vi "Tree_Sync_Hide items.vi"(7 "Action":T2, 8 "error in":errorcluster, 9 "Properties for Tree In":T1(array[cluster])=[{"Label"="AppBuilderCache", "Tag"="0.3.fa.AppBuilderCache", "Property Type"=enum."Base", "Indent"=0, "Can Read?"=FALSE, "Can Write?"=FALSE, "Is Read?"=FALSE, "Is Write?"=FALSE, "Inactive Parent?"=TRUE, "Unwired?"=FALSE}, {"Label"="Path", "Tag"="0.3.fa.AppBuilderCache:Path", "Property Type"=enum."Private", "Indent"=1, "Can Read?"=TRUE, "Can Write?"=FALSE, "Is Read?"=FALSE, "Is Write?"=FALSE, "Inactive Parent?"=FALSE, "Unwired?"=FALSE}, {"Label"="Application", "Tag"="1.2.80.Application", "Property Type"=enum."Base", "Indent"=0, "Can Read?"=FALSE, "Can Write?"=FALSE, "Is Read?"=FALSE, "Is Write?"=FALSE, "Inactive Parent?"=TRUE, "Unwired?"=FALSE}, {"Label"="Active", "Tag"="1.2.80.Application:Active", "Property Type"=enum."Base", "Indent"=1, "Can Read?"=FALSE, "Can Write?"=FALSE, "Is Read?"=FALSE, "Is Write?"=FALSE, "Inactive Parent?"=TRUE, "Unwired?"=FALSE}, {"Label"="Application", "Tag"="1.2.80.Application:Active:Application", "Property Type"=enum."Scripting", "Indent"=2, "Can Read?"=TRUE, "Can Write?"=FALSE, "Is Read?"=FALSE, "Is Write?"=FALSE, "Inactive Parent?"=FALSE, "Unwired?"=FALSE}, {"Label"="VI", "Tag"="2.2.46.Application:Active:VI", "Property Type"=enum."Scripting", "Indent"=2, "Can Read?"=TRUE, "Can Write?"=FALSE, "Is Read?"=FALSE, "Is Write?"=FALSE, "Inactive Parent?"=FALSE, "Unwired?"=FALSE}, {"Label"="All Contexts", "Tag"="3.3.68.Application:All Contexts", "Property Type"=enum."Private", "Indent"=1, "Can Read?"=TRUE, "Can Write?"=FALSE, "Is Read?"=FALSE, "Is Write?"=FALSE, "Inactive Parent?"=FALSE, "Unwired?"=FALSE}, {"Label"="All Libraries in Application Instance", "Tag"="4.1.cd.Application:All Libraries in Application Instance", "Property Type"=enum."Base", "Indent"=1, "Can Read?"=TRUE, "Can Write?"=FALSE, "Is Read?"=FALSE, "Is Write?"=FALSE, "Inactive Parent?"=FALSE, "Unwired?"=FALSE}, {"Label"="All System VIs in Memory", "Tag"="5.3.1e.Application:All System VIs in Memory", "Property Type"=enum."Private", "Indent"=1, "Can Read?"=TRUE, "Can Write?"=FALSE, "Is Read?"=FALSE, "Is Write?"=FALSE, "Inactive Parent?"=FALSE, "Unwired?"=FALSE}, {"Label"="All VIs In Memory", "Tag"="6.1.1c.Application:All VIs In Memory", "Property Type"=enum."Base", "Indent"=1, "Can Read?"=TRUE, "Can Write?"=FALSE, "Is Read?"=FALSE, "Is Write?"=FALSE, "Inactive Parent?"=FALSE, "Unwired?"=FALSE}, {"Label"="Assistants Use Strict Types Default", "Tag"="7.3.52.Application:Assistants Use Strict Types Default", "Property Type"=enum."Private", "Indent"=1, "Can Read?"=TRUE, "Can Write?"=TRUE, "Is Read?"=FALSE, "Is Write?"=FALSE, "Inactive Parent?"=FALSE, "Unwired?"=FALSE}, {"Label"="Auto-Route Wires", "Tag"="8.2.53.Application:Auto-Route Wires", "Property Type"=enum."Scripting", "Indent"=1, "Can Read?"=TRUE, "Can Write?"=TRUE, "Is Read?"=FALSE, "Is Write?"=FALSE, "Inactive Parent?"=FALSE, "Unwired?"=FALSE}, {"Label"="Available Environment Modes", "Tag"="9.3.dd.Application:Available Environment Modes", "Property Type"=enum."Private", "Indent"=1, "Can Read?"=TRUE, "Can Write?"=FALSE, "Is Read?"=FALSE, "Is Write?"=FALSE, "Inactive Parent?"=FALSE, "Unwired?"=FALSE}, {"Label"="Clipboard Mode", "Tag"="10.3.e4.Application:Clipboard Mode", "Property Type"=enum."Private", "Indent"=1, "Can Read?"=TRUE, "Can Write?"=TRUE, "Is Read?"=FALSE, "Is Write?"=FALSE, "Inactive Parent?"=FALSE, "Unwired?"=FALSE}, {"Label"="Clipboard VI", "Tag"="11.3.ad.Application:Clipboard VI", "Property Type"=enum."Private", "Indent"=1, "Can Read?"=TRUE, "Can Write?"=TRUE, "Is Read?"=FALSE, "Is Write?"=FALSE, "Inactive Parent?"=FALSE, "Unwired?"=FALSE}, {"Label"="Command Line Arguments", "Tag"="12.1.4f.Application:Command Line Arguments", "Property Type"=enum."Base", "Indent"=1, "Can Read?"=TRUE, "Can Write?"=FALSE, "Is Read?"=FALSE, "Is Write?"=FALSE, "Inactive Parent?"=FALSE, "Unwired?"=FALSE}, {"Label"="Compiler Threshold", "Tag"="13.2.fc.Application:Compiler Threshold", "Property Type"=enum."Scripting", "Indent"=1, "Can Read?"=TRUE, "Can Write?"=TRUE, "Is Read?"=FALSE, "Is Write?"=FALSE, "Inactive Parent?"=FALSE, "Unwired?"=FALSE}, {"Label"="Compiler", "Tag"="14.3.101.Application:Compiler", "Property Type"=enum."Base", "Indent"=1, "Can Read?"=FALSE, "Can Write?"=FALSE, "Is Read?"=FALSE, "Is Write?"=FALSE, "Inactive Parent?"=TRUE, "Unwired?"=FALSE}, {"Label"="AutoInlining", "Tag"="14.3.101.Application:Compiler:AutoInlining", "Property Type"=enum."Private", "Indent"=2, "Can Read?"=TRUE, "Can Write?"=TRUE, "Is Read?"=FALSE, "Is Write?"=FALSE, "Inactive Parent?"=FALSE, "Unwired?"=FALSE}, {"Label"="BriefDOT", "Tag"="15.3.d9.Application:Compiler:BriefDOT", "Property Type"=enum."Private", "Indent"=2, "Can Read?"=TRUE, "Can Write?"=TRUE, "Is Read?"=FALSE, "Is Write?"=FALSE, "Inactive Parent?"=FALSE, "Unwired?"=FALSE}, {"Label"="DFIR Compiler", "Tag"="16.3.af.Application:Compiler:DFIR Compiler", "Property Type"=enum."Private", "Indent"=2, "Can Read?"=TRUE, "Can Write?"=TRUE, "Is Read?"=FALSE, "Is Write?"=FALSE, "Inactive Parent?"=FALSE, "Unwired?"=FALSE}, {"Label"="DOT", "Tag"="17.3.c2.Application:Compiler:DOT", "Property Type"=enum."Private", "Indent"=2, "Can Read?"=TRUE, "Can Write?"=TRUE, "Is Read?"=FALSE, "Is Write?"=FALSE, "Inactive Parent?"=FALSE, "Unwired?"=FALSE}, {"Label"="FP Register Candidate", "Tag"="18.3.100.Application:Compiler:FP Register Candidate", "Property Type"=enum."Private", "Indent"=2, "Can Read?"=TRUE, "Can Write?"=TRUE, "Is Read?"=FALSE, "Is Write?"=FALSE, "Inactive Parent?"=FALSE, "Unwired?"=FALSE}, {"Label"="LLVM Compiler", "Tag"="19.3.ca.Application:Compiler:LLVM Compiler", "Property Type"=enum."Private", "Indent"=2, "Can Read?"=TRUE, "Can Write?"=TRUE, "Is Read?"=FALSE, "Is Write?"=FALSE, "Inactive Parent?"=FALSE, "Unwired?"=FALSE}, {"Label"="Sanity", "Tag"="20.3.c1.Application:Compiler:Sanity", "Property Type"=enum."Private", "Indent"=2, "Can Read?"=TRUE, "Can Write?"=TRUE, "Is Read?"=FALSE, "Is Write?"=FALSE, "Inactive Parent?"=FALSE, "Unwired?"=FALSE}, {"Label"="SSE Runtime Optimization", "Tag"="21.3.e6.Application:Compiler:SSE Runtime Optimization", "Property Type"=enum."Private", "Indent"=2, "Can Read?"=TRUE, "Can Write?"=TRUE, "Is Read?"=FALSE, "Is Write?"=FALSE, "Inactive Parent?"=FALSE, "Unwired?"=FALSE}, {"Label"="SSE1 Code Generation", "Tag"="22.3.ea.Application:Compiler:SSE1 Code Generation", "Property Type"=enum."Private", "Indent"=2, "Can Read?"=TRUE, "Can Write?"=TRUE, "Is Read?"=FALSE, "Is Write?"=FALSE, "Inactive Parent?"=FALSE, "Unwired?"=FALSE}, {"Label"="SSE2 Code Generation", "Tag"="23.3.eb.Application:Compiler:SSE2 Code Generation", "Property Type"=enum."Private", "Indent"=2, "Can Read?"=TRUE, "Can Write?"=TRUE, "Is Read?"=FALSE, "Is Write?"=FALSE, "Inactive Parent?"=FALSE, "Unwired?"=FALSE}, {"Label"="Context Name", "Tag"="24.3.7a.Application:Context Name", "Property Type"=enum."Private", "Indent"=1, "Can Read?"=TRUE, "Can Write?"=FALSE, "Is Read?"=FALSE, "Is Write?"=FALSE, "Inactive Parent?"=FALSE, "Unwired?"=FALSE}, {"Label"="Controls Palette Open", "Tag"="25.3.2a.Application:Controls Palette Open", "Property Type"=enum."Private", "Indent"=1, "Can Read?"=TRUE, "Can Write?"=TRUE, "Is Read?"=FALSE, "Is Write?"=FALSE, "Inactive Parent?"=FALSE, "Unwired?"=FALSE}, {"Label"="Cross Compile Count", "Tag"="26.3.fe.Application:Cross Compile Count", "Property Type"=enum."Private", "Indent"=1, "Can Read?"=TRUE, "Can Write?"=FALSE, "Is Read?"=FALSE, "Is Write?"=FALSE, "Inactive Parent?"=FALSE, "Unwired?"=FALSE}, {"Label"="Cross Context Settings", "Tag"="27.3.8e.Application:Cross Context Settings", "Property Type"=enum."Private", "Indent"=1, "Can Read?"=TRUE, "Can Write?"=FALSE, "Is Read?"=FALSE, "Is Write?"=FALSE, "Inactive Parent?"=FALSE, "Unwired?"=FALSE}, {"Label"="Current Environment Mode", "Tag"="28.1.ef.Application:Current Environment Mode", "Property Type"=enum."Base", "Indent"=1, "Can Read?"=TRUE, "Can Write?"=TRUE, "Is Read?"=FALSE, "Is Write?"=FALSE, "Inactive Parent?"=FALSE, "Unwired?"=FALSE}, {"Label"="Debug Name", "Tag"="29.1.8d.Application:Debug Name", "Property Type"=enum."Base", "Indent"=1, "Can Read?"=TRUE, "Can Write?"=FALSE, "Is Read?"=FALSE, "Is Write?"=FALSE, "Inactive Parent?"=FALSE, "Unwired?"=FALSE}, {"Label"="Default", "Tag"="30.1.90.Application:Default", "Property Type"=enum."Base", "Indent"=1, "Can Read?"=FALSE, "Can Write?"=FALSE, "Is Read?"=FALSE, "Is Write?"=FALSE, "Inactive Parent?"=TRUE, "Unwired?"=FALSE}, {"Label"="Application", "Tag"="30.1.90.Application:Default:Application", "Property Type"=enum."Base", "Indent"=2, "Can Read?"=TRUE, "Can Write?"=FALSE, "Is Read?"=FALSE, "Is Write?"=FALSE, "Inactive Parent?"=FALSE, "Unwired?"=FALSE}, {"Label"="Context Name", "Tag"="31.3.8f.Application:Default:Context Name", "Property Type"=enum."Private", "Indent"=2, "Can Read?"=TRUE, "Can Write?"=FALSE, "Is Read?"=FALSE, "Is Write?"=FALSE, "Inactive Parent?"=FALSE, "Unwired?"=FALSE}, {"Label"="Data Directory", "Tag"="32.1.57.Application:Default:Data Directory", "Property Type"=enum."Base", "Indent"=2, "Can Read?"=TRUE, "Can Write?"=FALSE, "Is Read?"=FALSE, "Is Write?"=FALSE, "Inactive Parent?"=FALSE, "Unwired?"=FALSE}, {"Label"="Error Handler VI", "Tag"="33.3.4e.Application:Default:Error Handler VI", "Property Type"=enum."Private", "Indent"=2, "Can Read?"=TRUE, "Can Write?"=TRUE, "Is Read?"=FALSE, "Is Write?"=FALSE, "Inactive Parent?"=FALSE, "Unwired?"=FALSE}, {"Label"="File Dialog Path", "Tag"="34.3.2d.Application:Default:File Dialog Path", "Property Type"=enum."Private", "Indent"=2, "Can Read?"=TRUE, "Can Write?"=TRUE, "Is Read?"=FALSE, "Is Write?"=FALSE, "Inactive Parent?"=FALSE, "Unwired?"=FALSE}, {"Label"="Defer Drawing", "Tag"="35.3.56.Application:Defer Drawing", "Property Type"=enum."Private", "Indent"=1, "Can Read?"=TRUE, "Can Write?"=TRUE, "Is Read?"=FALSE, "Is Write?"=FALSE, "Inactive Parent?"=FALSE, "Unwired?"=FALSE}, {"Label"="Delete FP Terminal from Diagram", "Tag"="36.2.5b.Application:Delete FP Terminal from Diagram", "Property Type"=enum."Scripting", "Indent"=1, "Can Read?"=TRUE, "Can Write?"=TRUE, "Is Read?"=FALSE, "Is Write?"=FALSE, "Inactive Parent?"=FALSE, "Unwired?"=FALSE}, {"Label"="Directory Path", "Tag"="37.1.19.Application:Directory Path", "Property Type"=enum."Base", "Indent"=1, "Can Read?"=TRUE, "Can Write?"=FALSE, "Is Read?"=FALSE, "Is Write?"=FALSE, "Inactive Parent?"=FALSE, "Unwired?"=FALSE}, {"Label"="Disable Path Case", "Tag"="38.3.e2.Application:Disable Path Case", "Property Type"=enum."Private", "Indent"=1, "Can Read?"=TRUE, "Can Write?"=TRUE, "Is Read?"=FALSE, "Is Write?"=FALSE, "Inactive Parent?"=FALSE, "Unwired?"=FALSE}, {"Label"="Downloaded VIs", "Tag"="39.3.3e.Application:Downloaded VIs", "Property Type"=enum."Private", "Indent"=1, "Can Read?"=TRUE, "Can Write?"=FALSE, "Is Read?"=FALSE, "Is Write?"=FALSE, "Inactive Parent?"=FALSE, "Unwired?"=FALSE}, {"Label"="DSC Support", "Tag"="40.3.ba.Application:DSC Support", "Property Type"=enum."Private", "Indent"=1, "Can Read?"=TRUE, "Can Write?"=FALSE, "Is Read?"=FALSE, "Is Write?"=FALSE, "Inactive Parent?"=FALSE, "Unwired?"=FALSE}, {"Label"="DWarn Dialog", "Tag"="41.3.6a.Application:DWarn Dialog", "Property Type"=enum."Private", "Indent"=1, "Can Read?"=TRUE, "Can Write?"=TRUE, "Is Read?"=FALSE, "Is Write?"=FALSE, "Inactive Parent?"=FALSE, "Unwired?"=FALSE}, {"Label"="Embedded Root Path", "Tag"="42.3.38.Application:Embedded Root Path", "Property Type"=enum."Private", "Indent"=1, "Can Read?"=TRUE, "Can Write?"=FALSE, "Is Read?"=FALSE, "Is Write?"=FALSE, "Inactive Parent?"=FALSE, "Unwired?"=FALSE}, {"Label"="Enable Binary Compatibility Load", "Tag"="43.3.111.Application:Enable Binary Compatibility Load", "Property Type"=enum."Private", "Indent"=1, "Can Read?"=TRUE, "Can Write?"=TRUE, "Is Read?"=FALSE, "Is Write?"=FALSE, "Inactive Parent?"=FALSE, "Unwired?"=FALSE}, {"Label"="Enable Inheritance LinkRef Addition", "Tag"="44.3.106.Application:Enable Inheritance LinkRef Addition", "Property Type"=enum."Private", "Indent"=1, "Can Read?"=TRUE, "Can Write?"=TRUE, "Is Read?"=FALSE, "Is Write?"=FALSE, "Inactive Parent?"=FALSE, "Unwired?"=FALSE}, {"Label"="Enable Inheritance LinkRefs", "Tag"="45.3.107.Application:Enable Inheritance LinkRefs", "Property Type"=enum."Private", "Indent"=1, "Can Read?"=TRUE, "Can Write?"=TRUE, "Is Read?"=FALSE, "Is Write?"=FALSE, "Inactive Parent?"=FALSE, "Unwired?"=FALSE}, {"Label"="EnableExcursionFreeExecSystems", "Tag"="46.3.112.Application:EnableExcursionFreeExecSystems", "Property Type"=enum."Private", "Indent"=1, "Can Read?"=TRUE, "Can Write?"=TRUE, "Is Read?"=FALSE, "Is Write?"=FALSE, "Inactive Parent?"=FALSE, "Unwired?"=FALSE}, {"Label"="Exported VIs In Memory", "Tag"="47.1.8.Application:Exported VIs In Memory", "Property Type"=enum."Base", "Indent"=1, "Can Read?"=TRUE, "Can Write?"=FALSE, "Is Read?"=FALSE, "Is Write?"=FALSE, "Inactive Parent?"=FALSE, "Unwired?"=FALSE}, {"Label"="Full Feature", "Tag"="48.3.67.Application:Full Feature", "Property Type"=enum."Private", "Indent"=1, "Can Read?"=TRUE, "Can Write?"=FALSE, "Is Read?"=FALSE, "Is Write?"=FALSE, "Inactive Parent?"=FALSE, "Unwired?"=FALSE}, {"Label"="Functions Palette Open", "Tag"="49.3.2b.Application:Functions Palette Open", "Property Type"=enum."Private", "Indent"=1, "Can Read?"=TRUE, "Can Write?"=TRUE, "Is Read?"=FALSE, "Is Write?"=FALSE, "Inactive Parent?"=FALSE, "Unwired?"=FALSE}, {"Label"="GdiCount", "Tag"="50.3.ff.Application:GdiCount", "Property Type"=enum."Private", "Indent"=1, "Can Read?"=TRUE, "Can Write?"=FALSE, "Is Read?"=FALSE, "Is Write?"=FALSE, "Inactive Parent?"=FALSE, "Unwired?"=FALSE}, {"Label"="Hide Load Warning", "Tag"="51.3.e1.Application:Hide Load Warning", "Property Type"=enum."Private", "Indent"=1, "Can Read?"=TRUE, "Can Write?"=TRUE, "Is Read?"=FALSE, "Is Write?"=FALSE, "Inactive Parent?"=FALSE, "Unwired?"=FALSE}, {"Label"="Host Preferences Section", "Tag"="52.3.3a.Application:Host Preferences Section", "Property Type"=enum."Private", "Indent"=1, "Can Read?"=TRUE, "Can Write?"=FALSE, "Is Read?"=FALSE, "Is Write?"=FALSE, "Inactive Parent?"=FALSE, "Unwired?"=FALSE}, {"Label"="IgnoreUnresolvedDLLRef", "Tag"="53.3.113.Application:IgnoreUnresolvedDLLRef", "Property Type"=enum."Private", "Indent"=1, "Can Read?"=TRUE, "Can Write?"=FALSE, "Is Read?"=FALSE, "Is Write?"=FALSE, "Inactive Parent?"=FALSE, "Unwired?"=FALSE}, {"Label"="ImageTableCount", "Tag"="54.3.114.Application:ImageTableCount", "Property Type"=enum."Private", "Indent"=1, "Can Read?"=TRUE, "Can Write?"=FALSE, "Is Read?"=FALSE, "Is Write?"=FALSE, "Inactive Parent?"=FALSE, "Unwired?"=FALSE}, {"Label"="ImageTableMaxCount", "Tag"="55.3.110.Application:ImageTableMaxCount", "Property Type"=enum."Private", "Indent"=1, "Can Read?"=TRUE, "Can Write?"=FALSE, "Is Read?"=FALSE, "Is Write?"=FALSE, "Inactive Parent?"=FALSE, "Unwired?"=FALSE}, {"Label"="Installed Package", "Tag"="56.3.5f.Application:Installed Package", "Property Type"=enum."Private", "Indent"=1, "Can Read?"=TRUE, "Can Write?"=FALSE, "Is Read?"=FALSE, "Is Write?"=FALSE, "Inactive Parent?"=FALSE, "Unwired?"=FALSE}, {"Label"="InstCachePath", "Tag"="57.3.f5.Application:InstCachePath", "Property Type"=enum."Private", "Indent"=1, "Can Read?"=TRUE, "Can Write?"=FALSE, "Is Read?"=FALSE, "Is Write?"=FALSE, "Inactive Parent?"=FALSE, "Unwired?"=FALSE}, {"Label"="Internet Toolkit Installed", "Tag"="58.3.62.Application:Internet Toolkit Installed", "Property Type"=enum."Private", "Indent"=1, "Can Read?"=TRUE, "Can Write?"=TRUE, "Is Read?"=FALSE, "Is Write?"=FALSE, "Inactive Parent?"=FALSE, "Unwired?"=FALSE}, {"Label"="Is Build App Instance", "Tag"="59.3.da.Application:Is Build App Instance", "Property Type"=enum."Private", "Indent"=1, "Can Read?"=TRUE, "Can Write?"=TRUE, "Is Read?"=FALSE, "Is Write?"=FALSE, "Inactive Parent?"=FALSE, "Unwired?"=FALSE}, {"Label"="Is Compile Suppressed", "Tag"="60.3.f6.Application:Is Compile Suppressed", "Property Type"=enum."Private", "Indent"=1, "Can Read?"=TRUE, "Can Write?"=TRUE, "Is Read?"=FALSE, "Is Write?"=FALSE, "Inactive Parent?"=FALSE, "Unwired?"=FALSE}, {"Label"="Is Editor In MDI Mode", "Tag"="61.3.7d.Application:Is Editor In MDI Mode", "Property Type"=enum."Private", "Indent"=1, "Can Read?"=TRUE, "Can Write?"=FALSE, "Is Read?"=FALSE, "Is Write?"=FALSE, "Inactive Parent?"=FALSE, "Unwired?"=FALSE}, {"Label"="Is Migration Enabled", "Tag"="62.3.a6.Application:Is Migration Enabled", "Property Type"=enum."Private", "Indent"=1, "Can Read?"=TRUE, "Can Write?"=TRUE, "Is Read?"=FALSE, "Is Write?"=FALSE, "Inactive Parent?"=FALSE, "Unwired?"=FALSE}, {"Label"="Kind", "Tag"="63.1.3.Application:Kind", "Property Type"=enum."Base", "Indent"=1, "Can Read?"=TRUE, "Can Write?"=FALSE, "Is Read?"=FALSE, "Is Write?"=FALSE, "Inactive Parent?"=FALSE, "Unwired?"=FALSE}, {"Label"="Language", "Tag"="64.1.63.Application:Language", "Property Type"=enum."Base", "Indent"=1, "Can Read?"=TRUE, "Can Write?"=FALSE, "Is Read?"=FALSE, "Is Write?"=FALSE, "Inactive Parent?"=FALSE, "Unwired?"=FALSE}, {"Label"="Legacy Build App File Layout", "Tag"="65.3.dc.Application:Legacy Build App File Layout", "Property Type"=enum."Private", "Indent"=1, "Can Read?"=TRUE, "Can Write?"=FALSE, "Is Read?"=FALSE, "Is Write?"=FALSE, "Inactive Parent?"=FALSE, "Unwired?"=FALSE}, {"Label"="Let Private Context Run With XNode", "Tag"="66.3.aa.Application:Let Private Context Run With XNode", "Property Type"=enum."Private", "Indent"=1, "Can Read?"=TRUE, "Can Write?"=TRUE, "Is Read?"=FALSE, "Is Write?"=FALSE, "Inactive Parent?"=FALSE, "Unwired?"=FALSE}, {"Label"="Library Finish Partial Load Enabled", "Tag"="67.3.f9.Application:Library Finish Partial Load Enabled", "Property Type"=enum."Private", "Indent"=1, "Can Read?"=TRUE, "Can Write?"=TRUE, "Is Read?"=FALSE, "Is Write?"=FALSE, "Inactive Parent?"=FALSE, "Unwired?"=FALSE}, {"Label"="Lock Instantiations for AppBuilder", "Tag"="68.3.e3.Application:Lock Instantiations for AppBuilder", "Property Type"=enum."Private", "Indent"=1, "Can Read?"=TRUE, "Can Write?"=TRUE, "Is Read?"=FALSE, "Is Write?"=FALSE, "Inactive Parent?"=FALSE, "Unwired?"=FALSE}, {"Label"="Locked Down For Build", "Tag"="69.3.fd.Application:Locked Down For Build", "Property Type"=enum."Private", "Indent"=1, "Can Read?"=TRUE, "Can Write?"=TRUE, "Is Read?"=FALSE, "Is Write?"=FALSE, "Inactive Parent?"=FALSE, "Unwired?"=FALSE}, {"Label"="LVTarget", "Tag"="70.3.83.Application:LVTarget", "Property Type"=enum."Private", "Indent"=1, "Can Read?"=TRUE, "Can Write?"=FALSE, "Is Read?"=FALSE, "Is Write?"=FALSE, "Inactive Parent?"=FALSE, "Unwired?"=FALSE}, {"Label"="Mass Compile Warn On Read Only VIs", "Tag"="71.3.f4.Application:Mass Compile Warn On Read Only VIs", "Property Type"=enum."Private", "Indent"=1, "Can Read?"=TRUE, "Can Write?"=TRUE, "Is Read?"=FALSE, "Is Write?"=FALSE, "Inactive Parent?"=FALSE, "Unwired?"=FALSE}, {"Label"="Menu Launch", "Tag"="72.2.7f.Application:Menu Launch", "Property Type"=enum."Base", "Indent"=1, "Can Read?"=FALSE, "Can Write?"=FALSE, "Is Read?"=FALSE, "Is Write?"=FALSE, "Inactive Parent?"=TRUE, "Unwired?"=FALSE}, {"Label"="App", "Tag"="72.2.7f.Application:Menu Launch:App", "Property Type"=enum."Scripting", "Indent"=2, "Can Read?"=TRUE, "Can Write?"=FALSE, "Is Read?"=FALSE, "Is Write?"=FALSE, "Inactive Parent?"=FALSE, "Unwired?"=FALSE}, {"Label"="VI", "Tag"="73.2.1d.Application:Menu Launch:VI", "Property Type"=enum."Scripting", "Indent"=2, "Can Read?"=TRUE, "Can Write?"=FALSE, "Is Read?"=FALSE, "Is Write?"=FALSE, "Inactive Parent?"=FALSE, "Unwired?"=FALSE}, {"Label"="Multi Pwd Op Cancelled?", "Tag"="74.3.a4.Application:Multi Pwd Op Cancelled?", "Property Type"=enum."Private", "Indent"=1, "Can Read?"=TRUE, "Can Write?"=FALSE, "Is Read?"=FALSE, "Is Write?"=FALSE, "Inactive Parent?"=FALSE, "Unwired?"=FALSE}, {"Label"="Name", "Tag"="75.1.0.Application:Name", "Property Type"=enum."Base", "Indent"=1, "Can Read?"=TRUE, "Can Write?"=FALSE, "Is Read?"=FALSE, "Is Write?"=FALSE, "Inactive Parent?"=FALSE, "Unwired?"=FALSE}, {"Label"="NativeEventTracingEnabled", "Tag"="76.3.118.Application:NativeEventTracingEnabled", "Property Type"=enum."Private", "Indent"=1, "Can Read?"=TRUE, "Can Write?"=TRUE, "Is Read?"=FALSE, "Is Write?"=FALSE, "Inactive Parent?"=FALSE, "Unwired?"=FALSE}, {"Label"="On Line", "Tag"="77.3.97.Application:On Line", "Property Type"=enum."Private", "Indent"=1, "Can Read?"=TRUE, "Can Write?"=TRUE, "Is Read?"=FALSE, "Is Write?"=FALSE, "Inactive Parent?"=FALSE, "Unwired?"=FALSE}, {"Label"="Parent Window For Dialogs", "Tag"="78.3.36.Application:Parent Window For Dialogs", "Property Type"=enum."Private", "Indent"=1, "Can Read?"=TRUE, "Can Write?"=TRUE, "Is Read?"=FALSE, "Is Write?"=FALSE, "Inactive Parent?"=FALSE, "Unwired?"=FALSE}, {"Label"="PPL LoadInCompatible LVVersion Default Value", "Tag"="79.3.115.Application:PPL LoadInCompatible LVVersion Default Value", "Property Type"=enum."Private", "Indent"=1, "Can Read?"=TRUE, "Can Write?"=TRUE, "Is Read?"=FALSE, "Is Write?"=FALSE, "Inactive Parent?"=FALSE, "Unwired?"=FALSE}, {"Label"="Preferences File Path", "Tag"="80.3.39.Application:Preferences File Path", "Property Type"=enum."Private", "Indent"=1, "Can Read?"=TRUE, "Can Write?"=FALSE, "Is Read?"=FALSE, "Is Write?"=FALSE, "Inactive Parent?"=FALSE, "Unwired?"=FALSE}, {"Label"="Private?", "Tag"="81.3.84.Application:Private?", "Property Type"=enum."Private", "Indent"=1, "Can Read?"=TRUE, "Can Write?"=FALSE, "Is Read?"=FALSE, "Is Write?"=FALSE, "Inactive Parent?"=FALSE, "Unwired?"=FALSE}, {"Label"="Property and Method Data Types", "Tag"="82.3.be.Application:Property and Method Data Types", "Property Type"=enum."Private", "Indent"=1, "Can Read?"=TRUE, "Can Write?"=FALSE, "Is Read?"=FALSE, "Is Write?"=FALSE, "Inactive Parent?"=FALSE, "Unwired?"=FALSE}, {"Label"="Pump OS Messages", "Tag"="83.3.66.Application:Pump OS Messages", "Property Type"=enum."Private", "Indent"=1, "Can Read?"=TRUE, "Can Write?"=TRUE, "Is Read?"=FALSE, "Is Write?"=FALSE, "Inactive Parent?"=FALSE, "Unwired?"=FALSE}, {"Label"="Real-Time Support", "Tag"="84.3.59.Application:Real-Time Support", "Property Type"=enum."Private", "Indent"=1, "Can Read?"=TRUE, "Can Write?"=FALSE, "Is Read?"=FALSE, "Is Write?"=FALSE, "Inactive Parent?"=FALSE, "Unwired?"=FALSE}, {"Label"="Registered Organization", "Tag"="85.3.3c.Application:Registered Organization", "Property Type"=enum."Private", "Indent"=1, "Can Read?"=TRUE, "Can Write?"=FALSE, "Is Read?"=FALSE, "Is Write?"=FALSE, "Inactive Parent?"=FALSE, "Unwired?"=FALSE}, {"Label"="Registered Owner", "Tag"="86.3.3b.Application:Registered Owner", "Property Type"=enum."Private", "Indent"=1, "Can Read?"=TRUE, "Can Write?"=FALSE, "Is Read?"=FALSE, "Is Write?"=FALSE, "Inactive Parent?"=FALSE, "Unwired?"=FALSE}, {"Label"="Remote Web Server Active", "Tag"="87.3.45.Application:Remote Web Server Active", "Property Type"=enum."Private", "Indent"=1, "Can Read?"=TRUE, "Can Write?"=FALSE, "Is Read?"=FALSE, "Is Write?"=FALSE, "Inactive Parent?"=FALSE, "Unwired?"=FALSE}, {"Label"="Rename Variables for AppBuilder", "Tag"="88.3.ed.Application:Rename Variables for AppBuilder", "Property Type"=enum."Private", "Indent"=1, "Can Read?"=TRUE, "Can Write?"=TRUE, "Is Read?"=FALSE, "Is Write?"=FALSE, "Inactive Parent?"=FALSE, "Unwired?"=FALSE}, {"Label"="Save Format", "Tag"="89.3.89.Application:Save Format", "Property Type"=enum."Private", "Indent"=1, "Can Read?"=TRUE, "Can Write?"=TRUE, "Is Read?"=FALSE, "Is Write?"=FALSE, "Inactive Parent?"=FALSE, "Unwired?"=FALSE}, {"Label"="Save Version", "Tag"="90.1.de.Application:Save Version", "Property Type"=enum."Base", "Indent"=1, "Can Read?"=TRUE, "Can Write?"=FALSE, "Is Read?"=FALSE, "Is Write?"=FALSE, "Inactive Parent?"=FALSE, "Unwired?"=FALSE}, {"Label"="Save Version As Integer", "Tag"="91.3.df.Application:Save Version As Integer", "Property Type"=enum."Private", "Indent"=1, "Can Read?"=TRUE, "Can Write?"=FALSE, "Is Read?"=FALSE, "Is Write?"=FALSE, "Inactive Parent?"=FALSE, "Unwired?"=FALSE}, {"Label"="Saveable Versions", "Tag"="92.1.b9.Application:Saveable Versions", "Property Type"=enum."Base", "Indent"=1, "Can Read?"=TRUE, "Can Write?"=FALSE, "Is Read?"=FALSE, "Is Write?"=FALSE, "Inactive Parent?"=FALSE, "Unwired?"=FALSE}, {"Label"="SaveChangesAutoSelection", "Tag"="93.3.117.Application:SaveChangesAutoSelection", "Property Type"=enum."Private", "Indent"=1, "Can Read?"=TRUE, "Can Write?"=TRUE, "Is Read?"=FALSE, "Is Write?"=FALSE, "Inactive Parent?"=FALSE, "Unwired?"=FALSE}, {"Label"="Search Paths", "Tag"="94.3.58.Application:Search Paths", "Property Type"=enum."Private", "Indent"=1, "Can Read?"=TRUE, "Can Write?"=TRUE, "Is Read?"=FALSE, "Is Write?"=FALSE, "Inactive Parent?"=FALSE, "Unwired?"=FALSE}, {"Label"="Selection List Changed", "Tag"="95.3.47.Application:Selection List Changed", "Property Type"=enum."Private", "Indent"=1, "Can Read?"=TRUE, "Can Write?"=FALSE, "Is Read?"=FALSE, "Is Write?"=FALSE, "Inactive Parent?"=FALSE, "Unwired?"=FALSE}, {"Label"="Selective Deallocation", "Tag"="96.3.103.Application:Selective Deallocation", "Property Type"=enum."Private", "Indent"=1, "Can Read?"=TRUE, "Can Write?"=TRUE, "Is Read?"=FALSE, "Is Write?"=FALSE, "Inactive Parent?"=FALSE, "Unwired?"=FALSE}, {"Label"="EnableForAllVIs", "Tag"="97.3.104.Application:Selective Deallocation:EnableForAllVIs", "Property Type"=enum."Private", "Indent"=2, "Can Read?"=TRUE, "Can Write?"=TRUE, "Is Read?"=FALSE, "Is Write?"=FALSE, "Inactive Parent?"=FALSE, "Unwired?"=FALSE}, {"Label"="LargeBufferThreshold", "Tag"="98.3.105.Application:Selective Deallocation:LargeBufferThreshold", "Property Type"=enum."Private", "Indent"=2, "Can Read?"=TRUE, "Can Write?"=TRUE, "Is Read?"=FALSE, "Is Write?"=FALSE, "Inactive Parent?"=FALSE, "Unwired?"=FALSE}, {"Label"="Serial Number", "Tag"="99.3.3d.Application:Serial Number", "Property Type"=enum."Private", "Indent"=1, "Can Read?"=TRUE, "Can Write?"=FALSE, "Is Read?"=FALSE, "Is Write?"=FALSE, "Inactive Parent?"=FALSE, "Unwired?"=FALSE}, {"Label"="Show FP Tip Strips", "Tag"="100.1.3f.Application:Show FP Tip Strips", "Property Type"=enum."Base", "Indent"=1, "Can Read?"=TRUE, "Can Write?"=TRUE, "Is Read?"=FALSE, "Is Write?"=FALSE, "Inactive Parent?"=FALSE, "Unwired?"=FALSE}, {"Label"="ShowAutoErrDialog", "Tag"="101.3.102.Application:ShowAutoErrDialog", "Property Type"=enum."Private", "Indent"=1, "Can Read?"=TRUE, "Can Write?"=TRUE, "Is Read?"=FALSE, "Is Write?"=FALSE, "Inactive Parent?"=FALSE, "Unwired?"=FALSE}, {"Label"="Target", "Tag"="102.3.8b.Application:Target", "Property Type"=enum."Base", "Indent"=1, "Can Read?"=FALSE, "Can Write?"=FALSE, "Is Read?"=FALSE, "Is Write?"=FALSE, "Inactive Parent?"=TRUE, "Unwired?"=FALSE}, {"Label"="Class Name", "Tag"="102.3.8b.Application:Target:Class Name", "Property Type"=enum."Private", "Indent"=2, "Can Read?"=TRUE, "Can Write?"=FALSE, "Is Read?"=FALSE, "Is Write?"=FALSE, "Inactive Parent?"=FALSE, "Unwired?"=FALSE}, {"Label"="CPU", "Tag"="103.1.5.Application:Target:CPU", "Property Type"=enum."Base", "Indent"=2, "Can Read?"=TRUE, "Can Write?"=FALSE, "Is Read?"=FALSE, "Is Write?"=FALSE, "Inactive Parent?"=FALSE, "Unwired?"=FALSE}, {"Label"="Current Processor ID", "Tag"="104.3.d2.Application:Target:Current Processor ID", "Property Type"=enum."Private", "Indent"=2, "Can Read?"=TRUE, "Can Write?"=FALSE, "Is Read?"=FALSE, "Is Write?"=FALSE, "Inactive Parent?"=FALSE, "Unwired?"=FALSE}, {"Label"="Data Cache Entry Sizes", "Tag"="105.1.d3.Application:Target:Data Cache Entry Sizes", "Property Type"=enum."Base", "Indent"=2, "Can Read?"=TRUE, "Can Write?"=FALSE, "Is Read?"=FALSE, "Is Write?"=FALSE, "Inactive Parent?"=FALSE, "Unwired?"=FALSE}, {"Label"="Data Cache Sizes", "Tag"="106.1.d4.Application:Target:Data Cache Sizes", "Property Type"=enum."Base", "Indent"=2, "Can Read?"=TRUE, "Can Write?"=FALSE, "Is Read?"=FALSE, "Is Write?"=FALSE, "Inactive Parent?"=FALSE, "Unwired?"=FALSE}, {"Label"="Info", "Tag"="107.3.54.Application:Target:Info", "Property Type"=enum."Private", "Indent"=2, "Can Read?"=TRUE, "Can Write?"=FALSE, "Is Read?"=FALSE, "Is Write?"=FALSE, "Inactive Parent?"=FALSE, "Unwired?"=FALSE}, {"Label"="IP Address", "Tag"="108.3.44.Application:Target:IP Address", "Property Type"=enum."Private", "Indent"=2, "Can Read?"=TRUE, "Can Write?"=FALSE, "Is Read?"=FALSE, "Is Write?"=FALSE, "Inactive Parent?"=FALSE, "Unwired?"=FALSE}, {"Label"="Number of Cores per Package", "Tag"="109.1.d0.Application:Target:Number of Cores per Package", "Property Type"=enum."Base", "Indent"=2, "Can Read?"=TRUE, "Can Write?"=FALSE, "Is Read?"=FALSE, "Is Write?"=FALSE, "Inactive Parent?"=FALSE, "Unwired?"=FALSE}, {"Label"="Number of Logical Processors", "Tag"="110.1.ce.Application:Target:Number of Logical Processors", "Property Type"=enum."Base", "Indent"=2, "Can Read?"=TRUE, "Can Write?"=FALSE, "Is Read?"=FALSE, "Is Write?"=FALSE, "Inactive Parent?"=FALSE, "Unwired?"=FALSE}, {"Label"="Number of Logical Processors per Core", "Tag"="111.1.d1.Application:Target:Number of Logical Processors per Core", "Property Type"=enum."Base", "Indent"=2, "Can Read?"=TRUE, "Can Write?"=FALSE, "Is Read?"=FALSE, "Is Write?"=FALSE, "Inactive Parent?"=FALSE, "Unwired?"=FALSE}, {"Label"="Number of Packages", "Tag"="112.1.d5.Application:Target:Number of Packages", "Property Type"=enum."Base", "Indent"=2, "Can Read?"=TRUE, "Can Write?"=FALSE, "Is Read?"=FALSE, "Is Write?"=FALSE, "Inactive Parent?"=FALSE, "Unwired?"=FALSE}, {"Label"="Operating System", "Tag"="113.1.4.Application:Target:Operating System", "Property Type"=enum."Base", "Indent"=2, "Can Read?"=TRUE, "Can Write?"=FALSE, "Is Read?"=FALSE, "Is Write?"=FALSE, "Inactive Parent?"=FALSE, "Unwired?"=FALSE}, {"Label"="TestStandOptions", "Tag"="114.3.db.Application:TestStandOptions", "Property Type"=enum."Private", "Indent"=1, "Can Read?"=TRUE, "Can Write?"=TRUE, "Is Read?"=FALSE, "Is Write?"=FALSE, "Inactive Parent?"=FALSE, "Unwired?"=FALSE}, {"Label"="Tools Palette Open", "Tag"="115.3.2c.Application:Tools Palette Open", "Property Type"=enum."Private", "Indent"=1, "Can Read?"=TRUE, "Can Write?"=TRUE, "Is Read?"=FALSE, "Is Write?"=FALSE, "Inactive Parent?"=FALSE, "Unwired?"=FALSE}, {"Label"="Treat LV 2016 As Binary Compatible", "Tag"="116.3.116.Application:Treat LV 2016 As Binary Compatible", "Property Type"=enum."Private", "Indent"=1, "Can Read?"=TRUE, "Can Write?"=TRUE, "Is Read?"=FALSE, "Is Write?"=FALSE, "Inactive Parent?"=FALSE, "Unwired?"=FALSE}, {"Label"="UD Refnum Files", "Tag"="117.3.ec.Application:UD Refnum Files", "Property Type"=enum."Private", "Indent"=1, "Can Read?"=TRUE, "Can Write?"=FALSE, "Is Read?"=FALSE, "Is Write?"=FALSE, "Inactive Parent?"=FALSE, "Unwired?"=FALSE}, {"Label"="Unattended Mode", "Tag"="118.3.4d.Application:Unattended Mode", "Property Type"=enum."Private", "Indent"=1, "Can Read?"=TRUE, "Can Write?"=TRUE, "Is Read?"=FALSE, "Is Write?"=FALSE, "Inactive Parent?"=FALSE, "Unwired?"=FALSE}, {"Label"="Use App Template Browser", "Tag"="119.3.51.Application:Use App Template Browser", "Property Type"=enum."Private", "Indent"=1, "Can Read?"=TRUE, "Can Write?"=TRUE, "Is Read?"=FALSE, "Is Write?"=FALSE, "Inactive Parent?"=FALSE, "Unwired?"=FALSE}, {"Label"="User Interface Available", "Tag"="120.1.5a.Application:User Interface Available", "Property Type"=enum."Base", "Indent"=1, "Can Read?"=TRUE, "Can Write?"=FALSE, "Is Read?"=FALSE, "Is Write?"=FALSE, "Inactive Parent?"=FALSE, "Unwired?"=FALSE}, {"Label"="User Name", "Tag"="121.1.1.Application:User Name", "Property Type"=enum."Base", "Indent"=1, "Can Read?"=TRUE, "Can Write?"=TRUE, "Is Read?"=FALSE, "Is Write?"=FALSE, "Inactive Parent?"=FALSE, "Unwired?"=FALSE}, {"Label"="Version As Integer", "Tag"="122.3.37.Application:Version As Integer", "Property Type"=enum."Private", "Indent"=1, "Can Read?"=TRUE, "Can Write?"=FALSE, "Is Read?"=FALSE, "Is Write?"=FALSE, "Inactive Parent?"=FALSE, "Unwired?"=FALSE}, {"Label"="Version Number", "Tag"="123.1.2.Application:Version Number", "Property Type"=enum."Base", "Indent"=1, "Can Read?"=TRUE, "Can Write?"=FALSE, "Is Read?"=FALSE, "Is Write?"=FALSE, "Inactive Parent?"=FALSE, "Unwired?"=FALSE}, {"Label"="Version Year", "Tag"="124.1.d7.Application:Version Year", "Property Type"=enum."Base", "Indent"=1, "Can Read?"=TRUE, "Can Write?"=FALSE, "Is Read?"=FALSE, "Is Write?"=FALSE, "Inactive Parent?"=FALSE, "Unwired?"=FALSE}, {"Label"="Version Year Number Only", "Tag"="125.3.109.Application:Version Year Number Only", "Property Type"=enum."Private", "Indent"=1, "Can Read?"=TRUE, "Can Write?"=FALSE, "Is Read?"=FALSE, "Is Write?"=FALSE, "Inactive Parent?"=FALSE, "Unwired?"=FALSE}, {"Label"="VI Of Top Most Block Diagram", "Tag"="126.2.9e.Application:VI Of Top Most Block Diagram", "Property Type"=enum."Scripting", "Indent"=1, "Can Read?"=TRUE, "Can Write?"=FALSE, "Is Read?"=FALSE, "Is Write?"=FALSE, "Inactive Parent?"=FALSE, "Unwired?"=FALSE}, {"Label"="Window For Panel Origin", "Tag"="127.3.64.Application:Window For Panel Origin", "Property Type"=enum."Private", "Indent"=1, "Can Read?"=TRUE, "Can Write?"=TRUE, "Is Read?"=FALSE, "Is Write?"=FALSE, "Inactive Parent?"=FALSE, "Unwired?"=FALSE}, {"Label"="Z Compress Level", "Tag"="128.3.96.Application:Z Compress Level", "Property Type"=enum."Private", "Indent"=1, "Can Read?"=TRUE, "Can Write?"=TRUE, "Is Read?"=FALSE, "Is Write?"=FALSE, "Inactive Parent?"=FALSE, "Unwired?"=FALSE}, {"Label"="Crosslink", "Tag"="129.3.a7.Crosslink", "Property Type"=enum."Base", "Indent"=0, "Can Read?"=FALSE, "Can Write?"=FALSE, "Is Read?"=FALSE, "Is Write?"=FALSE, "Inactive Parent?"=TRUE, "Unwired?"=FALSE}, {"Label"="Force Enable Dialogs", "Tag"="129.3.a7.Crosslink:Force Enable Dialogs", "Property Type"=enum."Private", "Indent"=1, "Can Read?"=TRUE, "Can Write?"=TRUE, "Is Read?"=FALSE, "Is Write?"=FALSE, "Inactive Parent?"=FALSE, "Unwired?"=FALSE}, {"Label"="Suppress Dialogs", "Tag"="130.3.a8.Crosslink:Suppress Dialogs", "Property Type"=enum."Private", "Indent"=1, "Can Read?"=TRUE, "Can Write?"=TRUE, "Is Read?"=FALSE, "Is Write?"=FALSE, "Inactive Parent?"=FALSE, "Unwired?"=FALSE}, {"Label"="Debug Server", "Tag"="131.1.98.Debug Server", "Property Type"=enum."Base", "Indent"=0, "Can Read?"=FALSE, "Can Write?"=FALSE, "Is Read?"=FALSE, "Is Write?"=FALSE, "Inactive Parent?"=TRUE, "Unwired?"=FALSE}, {"Label"="Server Active", "Tag"="131.1.98.Debug Server:Server Active", "Property Type"=enum."Base", "Indent"=1, "Can Read?"=TRUE, "Can Write?"=TRUE, "Is Read?"=FALSE, "Is Write?"=FALSE, "Inactive Parent?"=FALSE, "Unwired?"=FALSE}, {"Label"="TCP/IP Access List", "Tag"="132.1.99.Debug Server:TCP/IP Access List", "Property Type"=enum."Base", "Indent"=1, "Can Read?"=TRUE, "Can Write?"=TRUE, "Is Read?"=FALSE, "Is Write?"=FALSE, "Inactive Parent?"=FALSE, "Unwired?"=FALSE}, {"Label"="Delay File Notifications", "Tag"="133.3.a2.Delay File Notifications", "Property Type"=enum."Private", "Indent"=0, "Can Read?"=TRUE, "Can Write?"=TRUE, "Is Read?"=FALSE, "Is Write?"=FALSE, "Inactive Parent?"=FALSE, "Unwired?"=FALSE}, {"Label"="Display", "Tag"="134.1.22.Display", "Property Type"=enum."Base", "Indent"=0, "Can Read?"=FALSE, "Can Write?"=FALSE, "Is Read?"=FALSE, "Is Write?"=FALSE, "Inactive Parent?"=TRUE, "Unwired?"=FALSE}, {"Label"="All Monitors", "Tag"="134.1.22.Display:All Monitors", "Property Type"=enum."Base", "Indent"=1, "Can Read?"=TRUE, "Can Write?"=FALSE, "Is Read?"=FALSE, "Is Write?"=FALSE, "Inactive Parent?"=FALSE, "Unwired?"=FALSE}, {"Label"="Primary Workspace", "Tag"="135.1.21.Display:Primary Workspace", "Property Type"=enum."Base", "Indent"=1, "Can Read?"=TRUE, "Can Write?"=FALSE, "Is Read?"=FALSE, "Is Write?"=FALSE, "Inactive Parent?"=FALSE, "Unwired?"=FALSE}, {"Label"="Get NXT Context", "Tag"="136.3.e0.Get NXT Context", "Property Type"=enum."Private", "Indent"=0, "Can Read?"=TRUE, "Can Write?"=FALSE, "Is Read?"=FALSE, "Is Write?"=FALSE, "Inactive Parent?"=FALSE, "Unwired?"=FALSE}, {"Label"="Load and Save Warnings", "Tag"="137.3.bb.Load and Save Warnings", "Property Type"=enum."Base", "Indent"=0, "Can Read?"=FALSE, "Can Write?"=FALSE, "Is Read?"=FALSE, "Is Write?"=FALSE, "Inactive Parent?"=TRUE, "Unwired?"=FALSE}, {"Label"="Auto Test Mode", "Tag"="137.3.bb.Load and Save Warnings:Auto Test Mode", "Property Type"=enum."Private", "Indent"=1, "Can Read?"=TRUE, "Can Write?"=TRUE, "Is Read?"=FALSE, "Is Write?"=FALSE, "Inactive Parent?"=FALSE, "Unwired?"=FALSE}, {"Label"="History", "Tag"="138.3.bc.Load and Save Warnings:History", "Property Type"=enum."Private", "Indent"=1, "Can Read?"=TRUE, "Can Write?"=FALSE, "Is Read?"=FALSE, "Is Write?"=FALSE, "Inactive Parent?"=FALSE, "Unwired?"=FALSE}, {"Label"="MathScript", "Tag"="139.3.a5.MathScript", "Property Type"=enum."Base", "Indent"=0, "Can Read?"=FALSE, "Can Write?"=FALSE, "Is Read?"=FALSE, "Is Write?"=FALSE, "Inactive Parent?"=TRUE, "Unwired?"=FALSE}, {"Label"="All M Files In Context", "Tag"="139.3.a5.MathScript:All M Files In Context", "Property Type"=enum."Private", "Indent"=1, "Can Read?"=TRUE, "Can Write?"=FALSE, "Is Read?"=FALSE, "Is Write?"=FALSE, "Inactive Parent?"=FALSE, "Unwired?"=FALSE}, {"Label"="ColorsInSync", "Tag"="140.3.f1.MathScript:ColorsInSync", "Property Type"=enum."Private", "Indent"=1, "Can Read?"=TRUE, "Can Write?"=TRUE, "Is Read?"=FALSE, "Is Write?"=FALSE, "Inactive Parent?"=FALSE, "Unwired?"=FALSE}, {"Label"="Compiler Signature", "Tag"="141.3.e8.MathScript:Compiler Signature", "Property Type"=enum."Private", "Indent"=1, "Can Read?"=TRUE, "Can Write?"=FALSE, "Is Read?"=FALSE, "Is Write?"=FALSE, "Inactive Parent?"=FALSE, "Unwired?"=FALSE}, {"Label"="CompilerInMemory", "Tag"="142.3.f2.MathScript:CompilerInMemory", "Property Type"=enum."Private", "Indent"=1, "Can Read?"=TRUE, "Can Write?"=FALSE, "Is Read?"=FALSE, "Is Write?"=FALSE, "Inactive Parent?"=FALSE, "Unwired?"=FALSE}, {"Label"="HighlightingColors", "Tag"="143.3.f0.MathScript:HighlightingColors", "Property Type"=enum."Private", "Indent"=1, "Can Read?"=TRUE, "Can Write?"=FALSE, "Is Read?"=FALSE, "Is Write?"=FALSE, "Inactive Parent?"=FALSE, "Unwired?"=FALSE}, {"Label"="Path", "Tag"="144.3.a3.MathScript:Path", "Property Type"=enum."Private", "Indent"=1, "Can Read?"=TRUE, "Can Write?"=FALSE, "Is Read?"=FALSE, "Is Write?"=FALSE, "Inactive Parent?"=FALSE, "Unwired?"=FALSE}, {"Label"="Module Handle", "Tag"="145.3.65.Module Handle", "Property Type"=enum."Private", "Indent"=0, "Can Read?"=TRUE, "Can Write?"=FALSE, "Is Read?"=FALSE, "Is Write?"=FALSE, "Inactive Parent?"=FALSE, "Unwired?"=FALSE}, {"Label"="NI Security", "Tag"="146.1.a0.NI Security", "Property Type"=enum."Base", "Indent"=0, "Can Read?"=FALSE, "Can Write?"=FALSE, "Is Read?"=FALSE, "Is Write?"=FALSE, "Inactive Parent?"=TRUE, "Unwired?"=FALSE}, {"Label"="Nobody Logged In?", "Tag"="146.1.a0.NI Security:Nobody Logged In?", "Property Type"=enum."Base", "Indent"=1, "Can Read?"=TRUE, "Can Write?"=FALSE, "Is Read?"=FALSE, "Is Write?"=FALSE, "Inactive Parent?"=FALSE, "Unwired?"=FALSE}, {"Label"="Unique User", "Tag"="147.3.a1.NI Security:Unique User", "Property Type"=enum."Private", "Indent"=1, "Can Read?"=TRUE, "Can Write?"=FALSE, "Is Read?"=FALSE, "Is Write?"=FALSE, "Inactive Parent?"=FALSE, "Unwired?"=FALSE}, {"Label"="User", "Tag"="148.1.7c.NI Security:User", "Property Type"=enum."Base", "Indent"=1, "Can Read?"=TRUE, "Can Write?"=FALSE, "Is Read?"=FALSE, "Is Write?"=FALSE, "Inactive Parent?"=FALSE, "Unwired?"=FALSE}, {"Label"="Operating System", "Tag"="149.1.bf.Operating System", "Property Type"=enum."Base", "Indent"=0, "Can Read?"=FALSE, "Can Write?"=FALSE, "Is Read?"=FALSE, "Is Write?"=FALSE, "Inactive Parent?"=TRUE, "Unwired?"=FALSE}, {"Label"="Build Number", "Tag"="149.1.bf.Operating System:Build Number", "Property Type"=enum."Base", "Indent"=1, "Can Read?"=TRUE, "Can Write?"=FALSE, "Is Read?"=FALSE, "Is Write?"=FALSE, "Inactive Parent?"=FALSE, "Unwired?"=FALSE}, {"Label"="Detailed Name", "Tag"="150.1.c6.Operating System:Detailed Name", "Property Type"=enum."Base", "Indent"=1, "Can Read?"=TRUE, "Can Write?"=FALSE, "Is Read?"=FALSE, "Is Write?"=FALSE, "Inactive Parent?"=FALSE, "Unwired?"=FALSE}, {"Label"="Name", "Tag"="151.1.6.Operating System:Name", "Property Type"=enum."Base", "Indent"=1, "Can Read?"=TRUE, "Can Write?"=FALSE, "Is Read?"=FALSE, "Is Write?"=FALSE, "Inactive Parent?"=FALSE, "Unwired?"=FALSE}, {"Label"="Version Number", "Tag"="152.1.7.Operating System:Version Number", "Property Type"=enum."Base", "Indent"=1, "Can Read?"=TRUE, "Can Write?"=FALSE, "Is Read?"=FALSE, "Is Write?"=FALSE, "Inactive Parent?"=FALSE, "Unwired?"=FALSE}, {"Label"="Options", "Tag"="153.3.8c.Options", "Property Type"=enum."Base", "Indent"=0, "Can Read?"=FALSE, "Can Write?"=FALSE, "Is Read?"=FALSE, "Is Write?"=FALSE, "Inactive Parent?"=TRUE, "Unwired?"=FALSE}, {"Label"="Editor Menu Bar", "Tag"="153.3.8c.Options:Editor Menu Bar", "Property Type"=enum."Private", "Indent"=1, "Can Read?"=TRUE, "Can Write?"=FALSE, "Is Read?"=FALSE, "Is Write?"=FALSE, "Inactive Parent?"=FALSE, "Unwired?"=FALSE}, {"Label"="Use Abridged Menus", "Tag"="154.3.6b.Options:Use Abridged Menus", "Property Type"=enum."Private", "Indent"=1, "Can Read?"=TRUE, "Can Write?"=TRUE, "Is Read?"=FALSE, "Is Write?"=FALSE, "Inactive Parent?"=FALSE, "Unwired?"=FALSE}, {"Label"="Palettes", "Tag"="155.3.b2.Palettes", "Property Type"=enum."Base", "Indent"=0, "Can Read?"=FALSE, "Can Write?"=FALSE, "Is Read?"=FALSE, "Is Write?"=FALSE, "Inactive Parent?"=TRUE, "Unwired?"=FALSE}, {"Label"="Get Controls Names", "Tag"="155.3.b2.Palettes:Get Controls Names", "Property Type"=enum."Private", "Indent"=1, "Can Read?"=TRUE, "Can Write?"=FALSE, "Is Read?"=FALSE, "Is Write?"=FALSE, "Inactive Parent?"=FALSE, "Unwired?"=FALSE}, {"Label"="Get Functions Names", "Tag"="156.3.b1.Palettes:Get Functions Names", "Property Type"=enum."Private", "Indent"=1, "Can Read?"=TRUE, "Can Write?"=FALSE, "Is Read?"=FALSE, "Is Write?"=FALSE, "Inactive Parent?"=FALSE, "Unwired?"=FALSE}, {"Label"="Printing", "Tag"="157.1.4b.Printing", "Property Type"=enum."Base", "Indent"=0, "Can Read?"=FALSE, "Can Write?"=FALSE, "Is Read?"=FALSE, "Is Write?"=FALSE, "Inactive Parent?"=TRUE, "Unwired?"=FALSE}, {"Label"="Available Printers", "Tag"="157.1.4b.Printing:Available Printers", "Property Type"=enum."Base", "Indent"=1, "Can Read?"=TRUE, "Can Write?"=FALSE, "Is Read?"=FALSE, "Is Write?"=FALSE, "Inactive Parent?"=FALSE, "Unwired?"=FALSE}, {"Label"="Color/Grayscale?", "Tag"="158.1.48.Printing:Color/Grayscale?", "Property Type"=enum."Base", "Indent"=1, "Can Read?"=TRUE, "Can Write?"=TRUE, "Is Read?"=FALSE, "Is Write?"=FALSE, "Inactive Parent?"=FALSE, "Unwired?"=FALSE}, {"Label"="Custom All Controls?", "Tag"="159.1.29.Printing:Custom All Controls?", "Property Type"=enum."Base", "Indent"=1, "Can Read?"=TRUE, "Can Write?"=TRUE, "Is Read?"=FALSE, "Is Write?"=FALSE, "Inactive Parent?"=FALSE, "Unwired?"=FALSE}, {"Label"="Custom Cluster Constants?", "Tag"="160.1.e7.Printing:Custom Cluster Constants?", "Property Type"=enum."Base", "Indent"=1, "Can Read?"=TRUE, "Can Write?"=TRUE, "Is Read?"=FALSE, "Is Write?"=FALSE, "Inactive Parent?"=FALSE, "Unwired?"=FALSE}, {"Label"="Custom Connector?", "Tag"="161.1.c.Printing:Custom Connector?", "Property Type"=enum."Base", "Indent"=1, "Can Read?"=TRUE, "Can Write?"=TRUE, "Is Read?"=FALSE, "Is Write?"=FALSE, "Inactive Parent?"=FALSE, "Unwired?"=FALSE}, {"Label"="Custom Control Descriptions?", "Tag"="162.1.11.Printing:Custom Control Descriptions?", "Property Type"=enum."Base", "Indent"=1, "Can Read?"=TRUE, "Can Write?"=TRUE, "Is Read?"=FALSE, "Is Write?"=FALSE, "Inactive Parent?"=FALSE, "Unwired?"=FALSE}, {"Label"="Custom Control Label/Caption?", "Tag"="163.1.93.Printing:Custom Control Label/Caption?", "Property Type"=enum."Base", "Indent"=1, "Can Read?"=TRUE, "Can Write?"=TRUE, "Is Read?"=FALSE, "Is Write?"=FALSE, "Inactive Parent?"=FALSE, "Unwired?"=FALSE}, {"Label"="Custom Control Types?", "Tag"="164.1.12.Printing:Custom Control Types?", "Property Type"=enum."Base", "Indent"=1, "Can Read?"=TRUE, "Can Write?"=TRUE, "Is Read?"=FALSE, "Is Write?"=FALSE, "Inactive Parent?"=FALSE, "Unwired?"=FALSE}, {"Label"="Custom Controls?", "Tag"="165.1.10.Printing:Custom Controls?", "Property Type"=enum."Base", "Indent"=1, "Can Read?"=TRUE, "Can Write?"=TRUE, "Is Read?"=FALSE, "Is Write?"=FALSE, "Inactive Parent?"=FALSE, "Unwired?"=FALSE}, {"Label"="Custom Description?", "Tag"="166.1.d.Printing:Custom Description?", "Property Type"=enum."Base", "Indent"=1, "Can Read?"=TRUE, "Can Write?"=TRUE, "Is Read?"=FALSE, "Is Write?"=FALSE, "Inactive Parent?"=FALSE, "Unwired?"=FALSE}, {"Label"="Custom Diagram Hidden?", "Tag"="167.1.14.Printing:Custom Diagram Hidden?", "Property Type"=enum."Base", "Indent"=1, "Can Read?"=TRUE, "Can Write?"=TRUE, "Is Read?"=FALSE, "Is Write?"=FALSE, "Inactive Parent?"=FALSE, "Unwired?"=FALSE}, {"Label"="Custom Diagram Repeat?", "Tag"="168.1.15.Printing:Custom Diagram Repeat?", "Property Type"=enum."Base", "Indent"=1, "Can Read?"=TRUE, "Can Write?"=TRUE, "Is Read?"=FALSE, "Is Write?"=FALSE, "Inactive Parent?"=FALSE, "Unwired?"=FALSE}, {"Label"="Custom Diagram?", "Tag"="169.1.13.Printing:Custom Diagram?", "Property Type"=enum."Base", "Indent"=1, "Can Read?"=TRUE, "Can Write?"=TRUE, "Is Read?"=FALSE, "Is Write?"=FALSE, "Inactive Parent?"=FALSE, "Unwired?"=FALSE}, {"Label"="Custom Express VI Configuration?", "Tag"="170.1.5c.Printing:Custom Express VI Configuration?", "Property Type"=enum."Base", "Indent"=1, "Can Read?"=TRUE, "Can Write?"=TRUE, "Is Read?"=FALSE, "Is Write?"=FALSE, "Inactive Parent?"=FALSE, "Unwired?"=FALSE}, {"Label"="Custom Hierarchy?", "Tag"="171.1.17.Printing:Custom Hierarchy?", "Property Type"=enum."Base", "Indent"=1, "Can Read?"=TRUE, "Can Write?"=TRUE, "Is Read?"=FALSE, "Is Write?"=FALSE, "Inactive Parent?"=FALSE, "Unwired?"=FALSE}, {"Label"="Custom History?", "Tag"="172.1.18.Printing:Custom History?", "Property Type"=enum."Base", "Indent"=1, "Can Read?"=TRUE, "Can Write?"=TRUE, "Is Read?"=FALSE, "Is Write?"=FALSE, "Inactive Parent?"=FALSE, "Unwired?"=FALSE}, {"Label"="Custom List of SubVIs?", "Tag"="173.1.16.Printing:Custom List of SubVIs?", "Property Type"=enum."Base", "Indent"=1, "Can Read?"=TRUE, "Can Write?"=TRUE, "Is Read?"=FALSE, "Is Write?"=FALSE, "Inactive Parent?"=FALSE, "Unwired?"=FALSE}, {"Label"="Custom Panel Border?", "Tag"="174.1.f.Printing:Custom Panel Border?", "Property Type"=enum."Base", "Indent"=1, "Can Read?"=TRUE, "Can Write?"=TRUE, "Is Read?"=FALSE, "Is Write?"=FALSE, "Inactive Parent?"=FALSE, "Unwired?"=FALSE}, {"Label"="Custom Panel?", "Tag"="175.1.e.Printing:Custom Panel?", "Property Type"=enum."Base", "Indent"=1, "Can Read?"=TRUE, "Can Write?"=TRUE, "Is Read?"=FALSE, "Is Write?"=FALSE, "Inactive Parent?"=FALSE, "Unwired?"=FALSE}, {"Label"="Default Printer", "Tag"="176.1.49.Printing:Default Printer", "Property Type"=enum."Base", "Indent"=1, "Can Read?"=TRUE, "Can Write?"=TRUE, "Is Read?"=FALSE, "Is Write?"=FALSE, "Inactive Parent?"=FALSE, "Unwired?"=FALSE}, {"Label"="File Wrap Text Length", "Tag"="177.1.9.Printing:File Wrap Text Length", "Property Type"=enum."Base", "Indent"=1, "Can Read?"=TRUE, "Can Write?"=TRUE, "Is Read?"=FALSE, "Is Write?"=FALSE, "Inactive Parent?"=FALSE, "Unwired?"=FALSE}, {"Label"="JPEG Quality", "Tag"="178.1.b.Printing:JPEG Quality", "Property Type"=enum."Base", "Indent"=1, "Can Read?"=TRUE, "Can Write?"=TRUE, "Is Read?"=FALSE, "Is Write?"=FALSE, "Inactive Parent?"=FALSE, "Unwired?"=FALSE}, {"Label"="Method", "Tag"="179.1.4a.Printing:Method", "Property Type"=enum."Base", "Indent"=1, "Can Read?"=TRUE, "Can Write?"=TRUE, "Is Read?"=FALSE, "Is Write?"=FALSE, "Inactive Parent?"=FALSE, "Unwired?"=FALSE}, {"Label"="PNG Compression Level", "Tag"="180.1.a.Printing:PNG Compression Level", "Property Type"=enum."Base", "Indent"=1, "Can Read?"=TRUE, "Can Write?"=TRUE, "Is Read?"=FALSE, "Is Write?"=FALSE, "Inactive Parent?"=FALSE, "Unwired?"=FALSE}, {"Label"="Project", "Tag"="181.2.92.Project", "Property Type"=enum."Base", "Indent"=0, "Can Read?"=FALSE, "Can Write?"=FALSE, "Is Read?"=FALSE, "Is Write?"=FALSE, "Inactive Parent?"=TRUE, "Unwired?"=FALSE}, {"Label"="Active Project", "Tag"="181.2.92.Project:Active Project", "Property Type"=enum."Scripting", "Indent"=1, "Can Read?"=TRUE, "Can Write?"=FALSE, "Is Read?"=FALSE, "Is Write?"=FALSE, "Inactive Parent?"=FALSE, "Unwired?"=FALSE}, {"Label"="Default Project", "Tag"="182.3.81.Project:Default Project", "Property Type"=enum."Private", "Indent"=1, "Can Read?"=TRUE, "Can Write?"=FALSE, "Is Read?"=FALSE, "Is Write?"=FALSE, "Inactive Parent?"=FALSE, "Unwired?"=FALSE}, {"Label"="Get Last Max Load Time", "Tag"="183.3.87.Project:Get Last Max Load Time", "Property Type"=enum."Private", "Indent"=1, "Can Read?"=TRUE, "Can Write?"=FALSE, "Is Read?"=FALSE, "Is Write?"=FALSE, "Inactive Parent?"=FALSE, "Unwired?"=FALSE}, {"Label"="Has Any Project Been Created", "Tag"="184.3.82.Project:Has Any Project Been Created", "Property Type"=enum."Private", "Indent"=1, "Can Read?"=TRUE, "Can Write?"=FALSE, "Is Read?"=FALSE, "Is Write?"=FALSE, "Inactive Parent?"=FALSE, "Unwired?"=FALSE}, {"Label"="Libraries[]", "Tag"="185.3.88.Project:Libraries[]", "Property Type"=enum."Private", "Indent"=1, "Can Read?"=TRUE, "Can Write?"=FALSE, "Is Read?"=FALSE, "Is Write?"=FALSE, "Inactive Parent?"=FALSE, "Unwired?"=FALSE}, {"Label"="Owning Project", "Tag"="186.2.7e.Project:Owning Project", "Property Type"=enum."Scripting", "Indent"=1, "Can Read?"=TRUE, "Can Write?"=FALSE, "Is Read?"=FALSE, "Is Write?"=FALSE, "Inactive Parent?"=FALSE, "Unwired?"=FALSE}, {"Label"="Projects[]", "Tag"="187.1.69.Project:Projects[]", "Property Type"=enum."Base", "Indent"=1, "Can Read?"=TRUE, "Can Write?"=FALSE, "Is Read?"=FALSE, "Is Write?"=FALSE, "Inactive Parent?"=FALSE, "Unwired?"=FALSE}, {"Label"="Show Path in Project Window", "Tag"="188.3.85.Project:Show Path in Project Window", "Property Type"=enum."Private", "Indent"=1, "Can Read?"=TRUE, "Can Write?"=TRUE, "Is Read?"=FALSE, "Is Write?"=FALSE, "Inactive Parent?"=FALSE, "Unwired?"=FALSE}, {"Label"="Target Item", "Tag"="189.1.86.Project:Target Item", "Property Type"=enum."Base", "Indent"=1, "Can Read?"=TRUE, "Can Write?"=FALSE, "Is Read?"=FALSE, "Is Write?"=FALSE, "Inactive Parent?"=FALSE, "Unwired?"=FALSE}, {"Label"="Remote Panel", "Tag"="190.1.41.Remote Panel", "Property Type"=enum."Base", "Indent"=0, "Can Read?"=FALSE, "Can Write?"=FALSE, "Is Read?"=FALSE, "Is Write?"=FALSE, "Inactive Parent?"=TRUE, "Unwired?"=FALSE}, {"Label"="Connections To Clients", "Tag"="190.1.41.Remote Panel:Connections To Clients", "Property Type"=enum."Base", "Indent"=1, "Can Read?"=TRUE, "Can Write?"=FALSE, "Is Read?"=FALSE, "Is Write?"=FALSE, "Inactive Parent?"=FALSE, "Unwired?"=FALSE}, {"Label"="Connections To Servers", "Tag"="191.1.42.Remote Panel:Connections To Servers", "Property Type"=enum."Base", "Indent"=1, "Can Read?"=TRUE, "Can Write?"=FALSE, "Is Read?"=FALSE, "Is Write?"=FALSE, "Inactive Parent?"=FALSE, "Unwired?"=FALSE}, {"Label"="Is Supported", "Tag"="192.3.5e.Remote Panel:Is Supported", "Property Type"=enum."Private", "Indent"=1, "Can Read?"=TRUE, "Can Write?"=FALSE, "Is Read?"=FALSE, "Is Write?"=FALSE, "Inactive Parent?"=FALSE, "Unwired?"=FALSE}, {"Label"="NetLoad Monitor Enabled", "Tag"="193.3.43.Remote Panel:NetLoad Monitor Enabled", "Property Type"=enum."Private", "Indent"=1, "Can Read?"=TRUE, "Can Write?"=TRUE, "Is Read?"=FALSE, "Is Write?"=FALSE, "Inactive Parent?"=FALSE, "Unwired?"=FALSE}, {"Label"="Run Reserve XInterface Components", "Tag"="194.3.9f.Run Reserve XInterface Components", "Property Type"=enum."Private", "Indent"=0, "Can Read?"=TRUE, "Can Write?"=TRUE, "Is Read?"=FALSE, "Is Write?"=FALSE, "Inactive Parent?"=FALSE, "Unwired?"=FALSE}, {"Label"="Save for Previous", "Tag"="195.3.9d.Save for Previous", "Property Type"=enum."Base", "Indent"=0, "Can Read?"=FALSE, "Can Write?"=FALSE, "Is Read?"=FALSE, "Is Write?"=FALSE, "Inactive Parent?"=TRUE, "Unwired?"=FALSE}, {"Label"="Original App", "Tag"="195.3.9d.Save for Previous:Original App", "Property Type"=enum."Private", "Indent"=1, "Can Read?"=TRUE, "Can Write?"=FALSE, "Is Read?"=FALSE, "Is Write?"=FALSE, "Inactive Parent?"=FALSE, "Unwired?"=FALSE}, {"Label"="Separate Compiled Code For New Files", "Tag"="196.3.fb.Separate Compiled Code For New Files", "Property Type"=enum."Private", "Indent"=0, "Can Read?"=TRUE, "Can Write?"=FALSE, "Is Read?"=FALSE, "Is Write?"=FALSE, "Inactive Parent?"=FALSE, "Unwired?"=FALSE}, {"Label"="Server", "Tag"="197.1.27.Server", "Property Type"=enum."Base", "Indent"=0, "Can Read?"=FALSE, "Can Write?"=FALSE, "Is Read?"=FALSE, "Is Write?"=FALSE, "Inactive Parent?"=TRUE, "Unwired?"=FALSE}, {"Label"="Logging Enabled", "Tag"="197.1.27.Server:Logging Enabled", "Property Type"=enum."Base", "Indent"=1, "Can Read?"=TRUE, "Can Write?"=TRUE, "Is Read?"=FALSE, "Is Write?"=FALSE, "Inactive Parent?"=FALSE, "Unwired?"=FALSE}, {"Label"="Logging File Path", "Tag"="198.1.28.Server:Logging File Path", "Property Type"=enum."Base", "Indent"=1, "Can Read?"=TRUE, "Can Write?"=TRUE, "Is Read?"=FALSE, "Is Write?"=FALSE, "Inactive Parent?"=FALSE, "Unwired?"=FALSE}, {"Label"="Port", "Tag"="199.1.5d.Server:Port", "Property Type"=enum."Base", "Indent"=1, "Can Read?"=TRUE, "Can Write?"=TRUE, "Is Read?"=FALSE, "Is Write?"=FALSE, "Inactive Parent?"=FALSE, "Unwired?"=FALSE}, {"Label"="Service Name", "Tag"="200.1.94.Server:Service Name", "Property Type"=enum."Base", "Indent"=1, "Can Read?"=TRUE, "Can Write?"=TRUE, "Is Read?"=FALSE, "Is Write?"=FALSE, "Inactive Parent?"=FALSE, "Unwired?"=FALSE}, {"Label"="TCP Listener Active", "Tag"="201.1.20.Server:TCP Listener Active", "Property Type"=enum."Base", "Indent"=1, "Can Read?"=TRUE, "Can Write?"=TRUE, "Is Read?"=FALSE, "Is Write?"=FALSE, "Inactive Parent?"=FALSE, "Unwired?"=FALSE}, {"Label"="TCP/IP Access List", "Tag"="202.1.1b.Server:TCP/IP Access List", "Property Type"=enum."Base", "Indent"=1, "Can Read?"=TRUE, "Can Write?"=TRUE, "Is Read?"=FALSE, "Is Write?"=FALSE, "Inactive Parent?"=FALSE, "Unwired?"=FALSE}, {"Label"="VI Access List", "Tag"="203.1.1a.Server:VI Access List", "Property Type"=enum."Base", "Indent"=1, "Can Read?"=TRUE, "Can Write?"=TRUE, "Is Read?"=FALSE, "Is Write?"=FALSE, "Inactive Parent?"=FALSE, "Unwired?"=FALSE}, {"Label"="Source Control", "Tag"="204.3.6e.Source Control", "Property Type"=enum."Base", "Indent"=0, "Can Read?"=FALSE, "Can Write?"=FALSE, "Is Read?"=FALSE, "Is Write?"=FALSE, "Inactive Parent?"=TRUE, "Unwired?"=FALSE}, {"Label"="Configuration Data", "Tag"="204.3.6e.Source Control:Configuration Data", "Property Type"=enum."Private", "Indent"=1, "Can Read?"=TRUE, "Can Write?"=TRUE, "Is Read?"=FALSE, "Is Write?"=FALSE, "Inactive Parent?"=FALSE, "Unwired?"=FALSE}, {"Label"="Display Only Selected Files", "Tag"="205.3.71.Source Control:Display Only Selected Files", "Property Type"=enum."Private", "Indent"=1, "Can Read?"=TRUE, "Can Write?"=TRUE, "Is Read?"=FALSE, "Is Write?"=FALSE, "Inactive Parent?"=FALSE, "Unwired?"=FALSE}, {"Label"="Display Warning If File Is Checked Out", "Tag"="206.3.74.Source Control:Display Warning If File Is Checked Out", "Property Type"=enum."Private", "Indent"=1, "Can Read?"=TRUE, "Can Write?"=TRUE, "Is Read?"=FALSE, "Is Write?"=FALSE, "Inactive Parent?"=FALSE, "Unwired?"=FALSE}, {"Label"="Include InstrLib In Get Dependents", "Tag"="207.3.9c.Source Control:Include InstrLib In Get Dependents", "Property Type"=enum."Private", "Indent"=1, "Can Read?"=TRUE, "Can Write?"=TRUE, "Is Read?"=FALSE, "Is Write?"=FALSE, "Inactive Parent?"=FALSE, "Unwired?"=FALSE}, {"Label"="Include VILib In Get Dependents", "Tag"="208.3.9b.Source Control:Include VILib In Get Dependents", "Property Type"=enum."Private", "Indent"=1, "Can Read?"=TRUE, "Can Write?"=TRUE, "Is Read?"=FALSE, "Is Write?"=FALSE, "Inactive Parent?"=FALSE, "Unwired?"=FALSE}, {"Label"="Prompt to Add to SCC When Adding to Project", "Tag"="209.3.77.Source Control:Prompt to Add to SCC When Adding to Project", "Property Type"=enum."Private", "Indent"=1, "Can Read?"=TRUE, "Can Write?"=TRUE, "Is Read?"=FALSE, "Is Write?"=FALSE, "Inactive Parent?"=FALSE, "Unwired?"=FALSE}, {"Label"="Prompt to Check Out", "Tag"="210.3.76.Source Control:Prompt to Check Out", "Property Type"=enum."Private", "Indent"=1, "Can Read?"=TRUE, "Can Write?"=TRUE, "Is Read?"=FALSE, "Is Write?"=FALSE, "Inactive Parent?"=FALSE, "Unwired?"=FALSE}, {"Label"="Provider Location", "Tag"="211.3.70.Source Control:Provider Location", "Property Type"=enum."Private", "Indent"=1, "Can Read?"=TRUE, "Can Write?"=TRUE, "Is Read?"=FALSE, "Is Write?"=FALSE, "Inactive Parent?"=FALSE, "Unwired?"=FALSE}, {"Label"="Provider Name", "Tag"="212.3.6f.Source Control:Provider Name", "Property Type"=enum."Private", "Indent"=1, "Can Read?"=TRUE, "Can Write?"=TRUE, "Is Read?"=FALSE, "Is Write?"=FALSE, "Inactive Parent?"=FALSE, "Unwired?"=FALSE}, {"Label"="Select Callers When Checking Files Out", "Tag"="213.3.73.Source Control:Select Callers When Checking Files Out", "Property Type"=enum."Private", "Indent"=1, "Can Read?"=TRUE, "Can Write?"=TRUE, "Is Read?"=FALSE, "Is Write?"=FALSE, "Inactive Parent?"=FALSE, "Unwired?"=FALSE}, {"Label"="Select Hierarchy When Adding Files", "Tag"="214.3.72.Source Control:Select Hierarchy When Adding Files", "Property Type"=enum."Private", "Indent"=1, "Can Read?"=TRUE, "Can Write?"=TRUE, "Is Read?"=FALSE, "Is Write?"=FALSE, "Inactive Parent?"=FALSE, "Unwired?"=FALSE}, {"Label"="Use Dialog Box For File Checkout", "Tag"="215.3.75.Source Control:Use Dialog Box For File Checkout", "Property Type"=enum."Private", "Indent"=1, "Can Read?"=TRUE, "Can Write?"=TRUE, "Is Read?"=FALSE, "Is Write?"=FALSE, "Inactive Parent?"=FALSE, "Unwired?"=FALSE}, {"Label"="Statechart", "Tag"="216.3.b7.Statechart", "Property Type"=enum."Base", "Indent"=0, "Can Read?"=FALSE, "Can Write?"=FALSE, "Is Read?"=FALSE, "Is Write?"=FALSE, "Inactive Parent?"=TRUE, "Unwired?"=FALSE}, {"Label"="CodeGenCaseStruct", "Tag"="216.3.b7.Statechart:CodeGenCaseStruct", "Property Type"=enum."Private", "Indent"=1, "Can Read?"=TRUE, "Can Write?"=TRUE, "Is Read?"=FALSE, "Is Write?"=FALSE, "Inactive Parent?"=FALSE, "Unwired?"=FALSE}, {"Label"="InlineTopLevelGraph", "Tag"="217.3.bd.Statechart:InlineTopLevelGraph", "Property Type"=enum."Private", "Indent"=1, "Can Read?"=TRUE, "Can Write?"=TRUE, "Is Read?"=FALSE, "Is Write?"=FALSE, "Inactive Parent?"=FALSE, "Unwired?"=FALSE}, {"Label"="Is Installed", "Tag"="218.3.ee.Statechart:Is Installed", "Property Type"=enum."Private", "Indent"=1, "Can Read?"=TRUE, "Can Write?"=FALSE, "Is Read?"=FALSE, "Is Write?"=FALSE, "Inactive Parent?"=FALSE, "Unwired?"=FALSE}, {"Label"="Show Configuration", "Tag"="219.3.b4.Statechart:Show Configuration", "Property Type"=enum."Private", "Indent"=1, "Can Read?"=TRUE, "Can Write?"=FALSE, "Is Read?"=FALSE, "Is Write?"=FALSE, "Inactive Parent?"=FALSE, "Unwired?"=FALSE}, {"Label"="Show Custom Icon", "Tag"="220.3.b3.Statechart:Show Custom Icon", "Property Type"=enum."Private", "Indent"=1, "Can Read?"=TRUE, "Can Write?"=FALSE, "Is Read?"=FALSE, "Is Write?"=FALSE, "Inactive Parent?"=FALSE, "Unwired?"=FALSE}, {"Label"="Show Path for IsIn", "Tag"="221.3.b8.Statechart:Show Path for IsIn", "Property Type"=enum."Private", "Indent"=1, "Can Read?"=TRUE, "Can Write?"=FALSE, "Is Read?"=FALSE, "Is Write?"=FALSE, "Inactive Parent?"=FALSE, "Unwired?"=FALSE}, {"Label"="Suppress Auto Update Dependencies", "Tag"="222.3.a9.Suppress Auto Update Dependencies", "Property Type"=enum."Private", "Indent"=0, "Can Read?"=TRUE, "Can Write?"=TRUE, "Is Read?"=FALSE, "Is Write?"=FALSE, "Inactive Parent?"=FALSE, "Unwired?"=FALSE}, {"Label"="Supress Update Name Preflight", "Tag"="223.3.b0.Supress Update Name Preflight", "Property Type"=enum."Private", "Indent"=0, "Can Read?"=TRUE, "Can Write?"=TRUE, "Is Read?"=FALSE, "Is Write?"=FALSE, "Inactive Parent?"=FALSE, "Unwired?"=FALSE}, {"Label"="Tool Number", "Tag"="224.3.ae.Tool Number", "Property Type"=enum."Private", "Indent"=0, "Can Read?"=TRUE, "Can Write?"=TRUE, "Is Read?"=FALSE, "Is Write?"=FALSE, "Inactive Parent?"=FALSE, "Unwired?"=FALSE}, {"Label"="VIObjCache", "Tag"="225.3.f3.VIObjCache", "Property Type"=enum."Base", "Indent"=0, "Can Read?"=FALSE, "Can Write?"=FALSE, "Is Read?"=FALSE, "Is Write?"=FALSE, "Inactive Parent?"=TRUE, "Unwired?"=FALSE}, {"Label"="Available in RTE", "Tag"="225.3.f3.VIObjCache:Available in RTE", "Property Type"=enum."Private", "Indent"=1, "Can Read?"=TRUE, "Can Write?"=TRUE, "Is Read?"=FALSE, "Is Write?"=FALSE, "Inactive Parent?"=FALSE, "Unwired?"=FALSE}, {"Label"="DistPath", "Tag"="226.3.f7.VIObjCache:DistPath", "Property Type"=enum."Private", "Indent"=1, "Can Read?"=TRUE, "Can Write?"=FALSE, "Is Read?"=FALSE, "Is Write?"=FALSE, "Inactive Parent?"=FALSE, "Unwired?"=FALSE}, {"Label"="UserPath", "Tag"="227.3.f8.VIObjCache:UserPath", "Property Type"=enum."Private", "Indent"=1, "Can Read?"=TRUE, "Can Write?"=FALSE, "Is Read?"=FALSE, "Is Write?"=FALSE, "Inactive Parent?"=FALSE, "Unwired?"=FALSE}, {"Label"="Web Server", "Tag"="228.1.b5.Web Server", "Property Type"=enum."Base", "Indent"=0, "Can Read?"=FALSE, "Can Write?"=FALSE, "Is Read?"=FALSE, "Is Write?"=FALSE, "Inactive Parent?"=TRUE, "Unwired?"=FALSE}, {"Label"="Config File Path", "Tag"="228.1.b5.Web Server:Config File Path", "Property Type"=enum."Base", "Indent"=1, "Can Read?"=TRUE, "Can Write?"=FALSE, "Is Read?"=FALSE, "Is Write?"=FALSE, "Inactive Parent?"=FALSE, "Unwired?"=FALSE}, {"Label"="Default Config File Path", "Tag"="229.1.b6.Web Server:Default Config File Path", "Property Type"=enum."Base", "Indent"=1, "Can Read?"=TRUE, "Can Write?"=FALSE, "Is Read?"=FALSE, "Is Write?"=FALSE, "Inactive Parent?"=FALSE, "Unwired?"=FALSE}, {"Label"="HTTP Port", "Tag"="230.1.30.Web Server:HTTP Port", "Property Type"=enum."Base", "Indent"=1, "Can Read?"=TRUE, "Can Write?"=TRUE, "Is Read?"=FALSE, "Is Write?"=FALSE, "Inactive Parent?"=FALSE, "Unwired?"=FALSE}, {"Label"="Logging Enabled", "Tag"="231.1.32.Web Server:Logging Enabled", "Property Type"=enum."Base", "Indent"=1, "Can Read?"=TRUE, "Can Write?"=TRUE, "Is Read?"=FALSE, "Is Write?"=FALSE, "Inactive Parent?"=FALSE, "Unwired?"=FALSE}, {"Label"="Logging File Path", "Tag"="232.1.33.Web Server:Logging File Path", "Property Type"=enum."Base", "Indent"=1, "Can Read?"=TRUE, "Can Write?"=TRUE, "Is Read?"=FALSE, "Is Write?"=FALSE, "Inactive Parent?"=FALSE, "Unwired?"=FALSE}, {"Label"="Read Timeout", "Tag"="233.1.31.Web Server:Read Timeout", "Property Type"=enum."Base", "Indent"=1, "Can Read?"=TRUE, "Can Write?"=TRUE, "Is Read?"=FALSE, "Is Write?"=FALSE, "Inactive Parent?"=FALSE, "Unwired?"=FALSE}, {"Label"="Root Directory Path", "Tag"="234.1.2f.Web Server:Root Directory Path", "Property Type"=enum."Base", "Indent"=1, "Can Read?"=TRUE, "Can Write?"=TRUE, "Is Read?"=FALSE, "Is Write?"=FALSE, "Inactive Parent?"=FALSE, "Unwired?"=FALSE}, {"Label"="Server Active", "Tag"="235.1.2e.Web Server:Server Active", "Property Type"=enum."Base", "Indent"=1, "Can Read?"=TRUE, "Can Write?"=TRUE, "Is Read?"=FALSE, "Is Write?"=FALSE, "Inactive Parent?"=FALSE, "Unwired?"=FALSE}, {"Label"="TCP/IP Access List", "Tag"="236.1.34.Web Server:TCP/IP Access List", "Property Type"=enum."Base", "Indent"=1, "Can Read?"=TRUE, "Can Write?"=TRUE, "Is Read?"=FALSE, "Is Write?"=FALSE, "Inactive Parent?"=FALSE, "Unwired?"=FALSE}, {"Label"="VI Access List", "Tag"="237.1.35.Web Server:VI Access List", "Property Type"=enum."Base", "Indent"=1, "Can Read?"=TRUE, "Can Write?"=TRUE, "Is Read?"=FALSE, "Is Write?"=FALSE, "Inactive Parent?"=FALSE, "Unwired?"=FALSE}], 10 "Changed Tree Control Ref":refnum<vi>, 11 "All Tree Control Refs":refnum<vi>[](array[refnum])) -> (0 "error out":errorcluster)   [LabVIEW 2023]
uses:
  controls/action enum.ctl
panel:
  out "Properties for Tree with Value Update":T1(array[cluster])=[{"Label"="AppBuilderCache", "Tag"="0.3.fa.AppBuilderCache", "Property Type"=enum."Base", "Indent"=0, "Can Read?"=FALSE, "Can Write?"=FALSE, "Is Read?"=FALSE, "Is Write?"=FALSE, "Inactive Parent?"=TRUE, "Unwired?"=FALSE}, {"Label"="Path", "Tag"="0.3.fa.AppBuilderCache:Path", "Property Type"=enum."Private", "Indent"=1, "Can Read?"=TRUE, "Can Write?"=FALSE, "Is Read?"=FALSE, "Is Write?"=FALSE, "Inactive Parent?"=FALSE, "Unwired?"=FALSE}, {"Label"="Application", "Tag"="1.2.80.Application", "Property Type"=enum."Base", "Indent"=0, "Can Read?"=FALSE, "Can Write?"=FALSE, "Is Read?"=FALSE, "Is Write?"=FALSE, "Inactive Parent?"=TRUE, "Unwired?"=FALSE}, {"Label"="Active", "Tag"="1.2.80.Application:Active", "Property Type"=enum."Base", "Indent"=1, "Can Read?"=FALSE, "Can Write?"=FALSE, "Is Read?"=FALSE, "Is Write?"=FALSE, "Inactive Parent?"=TRUE, "Unwired?"=FALSE}, {"Label"="Application", "Tag"="1.2.80.Application:Active:Application", "Property Type"=enum."Scripting", "Indent"=2, "Can Read?"=TRUE, "Can Write?"=FALSE, "Is Read?"=FALSE, "Is Write?"=FALSE, "Inactive Parent?"=FALSE, "Unwired?"=FALSE}, {"Label"="VI", "Tag"="2.2.46.Application:Active:VI", "Property Type"=enum."Scripting", "Indent"=2, "Can Read?"=TRUE, "Can Write?"=FALSE, "Is Read?"=FALSE, "Is Write?"=FALSE, "Inactive Parent?"=FALSE, "Unwired?"=FALSE}, {"Label"="All Contexts", "Tag"="3.3.68.Application:All Contexts", "Property Type"=enum."Private", "Indent"=1, "Can Read?"=TRUE, "Can Write?"=FALSE, "Is Read?"=FALSE, "Is Write?"=FALSE, "Inactive Parent?"=FALSE, "Unwired?"=FALSE}, {"Label"="All Libraries in Application Instance", "Tag"="4.1.cd.Application:All Libraries in Application Instance", "Property Type"=enum."Base", "Indent"=1, "Can Read?"=TRUE, "Can Write?"=FALSE, "Is Read?"=FALSE, "Is Write?"=FALSE, "Inactive Parent?"=FALSE, "Unwired?"=FALSE}, {"Label"="All System VIs in Memory", "Tag"="5.3.1e.Application:All System VIs in Memory", "Property Type"=enum."Private", "Indent"=1, "Can Read?"=TRUE, "Can Write?"=FALSE, "Is Read?"=FALSE, "Is Write?"=FALSE, "Inactive Parent?"=FALSE, "Unwired?"=FALSE}, {"Label"="All VIs In Memory", "Tag"="6.1.1c.Application:All VIs In Memory", "Property Type"=enum."Base", "Indent"=1, "Can Read?"=TRUE, "Can Write?"=FALSE, "Is Read?"=FALSE, "Is Write?"=FALSE, "Inactive Parent?"=FALSE, "Unwired?"=FALSE}, {"Label"="Assistants Use Strict Types Default", "Tag"="7.3.52.Application:Assistants Use Strict Types Default", "Property Type"=enum."Private", "Indent"=1, "Can Read?"=TRUE, "Can Write?"=TRUE, "Is Read?"=FALSE, "Is Write?"=FALSE, "Inactive Parent?"=FALSE, "Unwired?"=FALSE}, {"Label"="Auto-Route Wires", "Tag"="8.2.53.Application:Auto-Route Wires", "Property Type"=enum."Scripting", "Indent"=1, "Can Read?"=TRUE, "Can Write?"=TRUE, "Is Read?"=FALSE, "Is Write?"=FALSE, "Inactive Parent?"=FALSE, "Unwired?"=FALSE}, {"Label"="Available Environment Modes", "Tag"="9.3.dd.Application:Available Environment Modes", "Property Type"=enum."Private", "Indent"=1, "Can Read?"=TRUE, "Can Write?"=FALSE, "Is Read?"=FALSE, "Is Write?"=FALSE, "Inactive Parent?"=FALSE, "Unwired?"=FALSE}, {"Label"="Clipboard Mode", "Tag"="10.3.e4.Application:Clipboard Mode", "Property Type"=enum."Private", "Indent"=1, "Can Read?"=TRUE, "Can Write?"=TRUE, "Is Read?"=FALSE, "Is Write?"=FALSE, "Inactive Parent?"=FALSE, "Unwired?"=FALSE}, {"Label"="Clipboard VI", "Tag"="11.3.ad.Application:Clipboard VI", "Property Type"=enum."Private", "Indent"=1, "Can Read?"=TRUE, "Can Write?"=TRUE, "Is Read?"=FALSE, "Is Write?"=FALSE, "Inactive Parent?"=FALSE, "Unwired?"=FALSE}, {"Label"="Command Line Arguments", "Tag"="12.1.4f.Application:Command Line Arguments", "Property Type"=enum."Base", "Indent"=1, "Can Read?"=TRUE, "Can Write?"=FALSE, "Is Read?"=FALSE, "Is Write?"=FALSE, "Inactive Parent?"=FALSE, "Unwired?"=FALSE}, {"Label"="Compiler Threshold", "Tag"="13.2.fc.Application:Compiler Threshold", "Property Type"=enum."Scripting", "Indent"=1, "Can Read?"=TRUE, "Can Write?"=TRUE, "Is Read?"=FALSE, "Is Write?"=FALSE, "Inactive Parent?"=FALSE, "Unwired?"=FALSE}, {"Label"="Compiler", "Tag"="14.3.101.Application:Compiler", "Property Type"=enum."Base", "Indent"=1, "Can Read?"=FALSE, "Can Write?"=FALSE, "Is Read?"=FALSE, "Is Write?"=FALSE, "Inactive Parent?"=TRUE, "Unwired?"=FALSE}, {"Label"="AutoInlining", "Tag"="14.3.101.Application:Compiler:AutoInlining", "Property Type"=enum."Private", "Indent"=2, "Can Read?"=TRUE, "Can Write?"=TRUE, "Is Read?"=FALSE, "Is Write?"=FALSE, "Inactive Parent?"=FALSE, "Unwired?"=FALSE}, {"Label"="BriefDOT", "Tag"="15.3.d9.Application:Compiler:BriefDOT", "Property Type"=enum."Private", "Indent"=2, "Can Read?"=TRUE, "Can Write?"=TRUE, "Is Read?"=FALSE, "Is Write?"=FALSE, "Inactive Parent?"=FALSE, "Unwired?"=FALSE}, {"Label"="DFIR Compiler", "Tag"="16.3.af.Application:Compiler:DFIR Compiler", "Property Type"=enum."Private", "Indent"=2, "Can Read?"=TRUE, "Can Write?"=TRUE, "Is Read?"=FALSE, "Is Write?"=FALSE, "Inactive Parent?"=FALSE, "Unwired?"=FALSE}, {"Label"="DOT", "Tag"="17.3.c2.Application:Compiler:DOT", "Property Type"=enum."Private", "Indent"=2, "Can Read?"=TRUE, "Can Write?"=TRUE, "Is Read?"=FALSE, "Is Write?"=FALSE, "Inactive Parent?"=FALSE, "Unwired?"=FALSE}, {"Label"="FP Register Candidate", "Tag"="18.3.100.Application:Compiler:FP Register Candidate", "Property Type"=enum."Private", "Indent"=2, "Can Read?"=TRUE, "Can Write?"=TRUE, "Is Read?"=FALSE, "Is Write?"=FALSE, "Inactive Parent?"=FALSE, "Unwired?"=FALSE}, {"Label"="LLVM Compiler", "Tag"="19.3.ca.Application:Compiler:LLVM Compiler", "Property Type"=enum."Private", "Indent"=2, "Can Read?"=TRUE, "Can Write?"=TRUE, "Is Read?"=FALSE, "Is Write?"=FALSE, "Inactive Parent?"=FALSE, "Unwired?"=FALSE}, {"Label"="Sanity", "Tag"="20.3.c1.Application:Compiler:Sanity", "Property Type"=enum."Private", "Indent"=2, "Can Read?"=TRUE, "Can Write?"=TRUE, "Is Read?"=FALSE, "Is Write?"=FALSE, "Inactive Parent?"=FALSE, "Unwired?"=FALSE}, {"Label"="SSE Runtime Optimization", "Tag"="21.3.e6.Application:Compiler:SSE Runtime Optimization", "Property Type"=enum."Private", "Indent"=2, "Can Read?"=TRUE, "Can Write?"=TRUE, "Is Read?"=FALSE, "Is Write?"=FALSE, "Inactive Parent?"=FALSE, "Unwired?"=FALSE}, {"Label"="SSE1 Code Generation", "Tag"="22.3.ea.Application:Compiler:SSE1 Code Generation", "Property Type"=enum."Private", "Indent"=2, "Can Read?"=TRUE, "Can Write?"=TRUE, "Is Read?"=FALSE, "Is Write?"=FALSE, "Inactive Parent?"=FALSE, "Unwired?"=FALSE}, {"Label"="SSE2 Code Generation", "Tag"="23.3.eb.Application:Compiler:SSE2 Code Generation", "Property Type"=enum."Private", "Indent"=2, "Can Read?"=TRUE, "Can Write?"=TRUE, "Is Read?"=FALSE, "Is Write?"=FALSE, "Inactive Parent?"=FALSE, "Unwired?"=FALSE}, {"Label"="Context Name", "Tag"="24.3.7a.Application:Context Name", "Property Type"=enum."Private", "Indent"=1, "Can Read?"=TRUE, "Can Write?"=FALSE, "Is Read?"=FALSE, "Is Write?"=FALSE, "Inactive Parent?"=FALSE, "Unwired?"=FALSE}, {"Label"="Controls Palette Open", "Tag"="25.3.2a.Application:Controls Palette Open", "Property Type"=enum."Private", "Indent"=1, "Can Read?"=TRUE, "Can Write?"=TRUE, "Is Read?"=FALSE, "Is Write?"=FALSE, "Inactive Parent?"=FALSE, "Unwired?"=FALSE}, {"Label"="Cross Compile Count", "Tag"="26.3.fe.Application:Cross Compile Count", "Property Type"=enum."Private", "Indent"=1, "Can Read?"=TRUE, "Can Write?"=FALSE, "Is Read?"=FALSE, "Is Write?"=FALSE, "Inactive Parent?"=FALSE, "Unwired?"=FALSE}, {"Label"="Cross Context Settings", "Tag"="27.3.8e.Application:Cross Context Settings", "Property Type"=enum."Private", "Indent"=1, "Can Read?"=TRUE, "Can Write?"=FALSE, "Is Read?"=FALSE, "Is Write?"=FALSE, "Inactive Parent?"=FALSE, "Unwired?"=FALSE}, {"Label"="Current Environment Mode", "Tag"="28.1.ef.Application:Current Environment Mode", "Property Type"=enum."Base", "Indent"=1, "Can Read?"=TRUE, "Can Write?"=TRUE, "Is Read?"=FALSE, "Is Write?"=FALSE, "Inactive Parent?"=FALSE, "Unwired?"=FALSE}, {"Label"="Debug Name", "Tag"="29.1.8d.Application:Debug Name", "Property Type"=enum."Base", "Indent"=1, "Can Read?"=TRUE, "Can Write?"=FALSE, "Is Read?"=FALSE, "Is Write?"=FALSE, "Inactive Parent?"=FALSE, "Unwired?"=FALSE}, {"Label"="Default", "Tag"="30.1.90.Application:Default", "Property Type"=enum."Base", "Indent"=1, "Can Read?"=FALSE, "Can Write?"=FALSE, "Is Read?"=FALSE, "Is Write?"=FALSE, "Inactive Parent?"=TRUE, "Unwired?"=FALSE}, {"Label"="Application", "Tag"="30.1.90.Application:Default:Application", "Property Type"=enum."Base", "Indent"=2, "Can Read?"=TRUE, "Can Write?"=FALSE, "Is Read?"=FALSE, "Is Write?"=FALSE, "Inactive Parent?"=FALSE, "Unwired?"=FALSE}, {"Label"="Context Name", "Tag"="31.3.8f.Application:Default:Context Name", "Property Type"=enum."Private", "Indent"=2, "Can Read?"=TRUE, "Can Write?"=FALSE, "Is Read?"=FALSE, "Is Write?"=FALSE, "Inactive Parent?"=FALSE, "Unwired?"=FALSE}, {"Label"="Data Directory", "Tag"="32.1.57.Application:Default:Data Directory", "Property Type"=enum."Base", "Indent"=2, "Can Read?"=TRUE, "Can Write?"=FALSE, "Is Read?"=FALSE, "Is Write?"=FALSE, "Inactive Parent?"=FALSE, "Unwired?"=FALSE}, {"Label"="Error Handler VI", "Tag"="33.3.4e.Application:Default:Error Handler VI", "Property Type"=enum."Private", "Indent"=2, "Can Read?"=TRUE, "Can Write?"=TRUE, "Is Read?"=FALSE, "Is Write?"=FALSE, "Inactive Parent?"=FALSE, "Unwired?"=FALSE}, {"Label"="File Dialog Path", "Tag"="34.3.2d.Application:Default:File Dialog Path", "Property Type"=enum."Private", "Indent"=2, "Can Read?"=TRUE, "Can Write?"=TRUE, "Is Read?"=FALSE, "Is Write?"=FALSE, "Inactive Parent?"=FALSE, "Unwired?"=FALSE}, {"Label"="Defer Drawing", "Tag"="35.3.56.Application:Defer Drawing", "Property Type"=enum."Private", "Indent"=1, "Can Read?"=TRUE, "Can Write?"=TRUE, "Is Read?"=FALSE, "Is Write?"=FALSE, "Inactive Parent?"=FALSE, "Unwired?"=FALSE}, {"Label"="Delete FP Terminal from Diagram", "Tag"="36.2.5b.Application:Delete FP Terminal from Diagram", "Property Type"=enum."Scripting", "Indent"=1, "Can Read?"=TRUE, "Can Write?"=TRUE, "Is Read?"=FALSE, "Is Write?"=FALSE, "Inactive Parent?"=FALSE, "Unwired?"=FALSE}, {"Label"="Directory Path", "Tag"="37.1.19.Application:Directory Path", "Property Type"=enum."Base", "Indent"=1, "Can Read?"=TRUE, "Can Write?"=FALSE, "Is Read?"=FALSE, "Is Write?"=FALSE, "Inactive Parent?"=FALSE, "Unwired?"=FALSE}, {"Label"="Disable Path Case", "Tag"="38.3.e2.Application:Disable Path Case", "Property Type"=enum."Private", "Indent"=1, "Can Read?"=TRUE, "Can Write?"=TRUE, "Is Read?"=FALSE, "Is Write?"=FALSE, "Inactive Parent?"=FALSE, "Unwired?"=FALSE}, {"Label"="Downloaded VIs", "Tag"="39.3.3e.Application:Downloaded VIs", "Property Type"=enum."Private", "Indent"=1, "Can Read?"=TRUE, "Can Write?"=FALSE, "Is Read?"=FALSE, "Is Write?"=FALSE, "Inactive Parent?"=FALSE, "Unwired?"=FALSE}, {"Label"="DSC Support", "Tag"="40.3.ba.Application:DSC Support", "Property Type"=enum."Private", "Indent"=1, "Can Read?"=TRUE, "Can Write?"=FALSE, "Is Read?"=FALSE, "Is Write?"=FALSE, "Inactive Parent?"=FALSE, "Unwired?"=FALSE}, {"Label"="DWarn Dialog", "Tag"="41.3.6a.Application:DWarn Dialog", "Property Type"=enum."Private", "Indent"=1, "Can Read?"=TRUE, "Can Write?"=TRUE, "Is Read?"=FALSE, "Is Write?"=FALSE, "Inactive Parent?"=FALSE, "Unwired?"=FALSE}, {"Label"="Embedded Root Path", "Tag"="42.3.38.Application:Embedded Root Path", "Property Type"=enum."Private", "Indent"=1, "Can Read?"=TRUE, "Can Write?"=FALSE, "Is Read?"=FALSE, "Is Write?"=FALSE, "Inactive Parent?"=FALSE, "Unwired?"=FALSE}, {"Label"="Enable Binary Compatibility Load", "Tag"="43.3.111.Application:Enable Binary Compatibility Load", "Property Type"=enum."Private", "Indent"=1, "Can Read?"=TRUE, "Can Write?"=TRUE, "Is Read?"=FALSE, "Is Write?"=FALSE, "Inactive Parent?"=FALSE, "Unwired?"=FALSE}, {"Label"="Enable Inheritance LinkRef Addition", "Tag"="44.3.106.Application:Enable Inheritance LinkRef Addition", "Property Type"=enum."Private", "Indent"=1, "Can Read?"=TRUE, "Can Write?"=TRUE, "Is Read?"=FALSE, "Is Write?"=FALSE, "Inactive Parent?"=FALSE, "Unwired?"=FALSE}, {"Label"="Enable Inheritance LinkRefs", "Tag"="45.3.107.Application:Enable Inheritance LinkRefs", "Property Type"=enum."Private", "Indent"=1, "Can Read?"=TRUE, "Can Write?"=TRUE, "Is Read?"=FALSE, "Is Write?"=FALSE, "Inactive Parent?"=FALSE, "Unwired?"=FALSE}, {"Label"="EnableExcursionFreeExecSystems", "Tag"="46.3.112.Application:EnableExcursionFreeExecSystems", "Property Type"=enum."Private", "Indent"=1, "Can Read?"=TRUE, "Can Write?"=TRUE, "Is Read?"=FALSE, "Is Write?"=FALSE, "Inactive Parent?"=FALSE, "Unwired?"=FALSE}, {"Label"="Exported VIs In Memory", "Tag"="47.1.8.Application:Exported VIs In Memory", "Property Type"=enum."Base", "Indent"=1, "Can Read?"=TRUE, "Can Write?"=FALSE, "Is Read?"=FALSE, "Is Write?"=FALSE, "Inactive Parent?"=FALSE, "Unwired?"=FALSE}, {"Label"="Full Feature", "Tag"="48.3.67.Application:Full Feature", "Property Type"=enum."Private", "Indent"=1, "Can Read?"=TRUE, "Can Write?"=FALSE, "Is Read?"=FALSE, "Is Write?"=FALSE, "Inactive Parent?"=FALSE, "Unwired?"=FALSE}, {"Label"="Functions Palette Open", "Tag"="49.3.2b.Application:Functions Palette Open", "Property Type"=enum."Private", "Indent"=1, "Can Read?"=TRUE, "Can Write?"=TRUE, "Is Read?"=FALSE, "Is Write?"=FALSE, "Inactive Parent?"=FALSE, "Unwired?"=FALSE}, {"Label"="GdiCount", "Tag"="50.3.ff.Application:GdiCount", "Property Type"=enum."Private", "Indent"=1, "Can Read?"=TRUE, "Can Write?"=FALSE, "Is Read?"=FALSE, "Is Write?"=FALSE, "Inactive Parent?"=FALSE, "Unwired?"=FALSE}, {"Label"="Hide Load Warning", "Tag"="51.3.e1.Application:Hide Load Warning", "Property Type"=enum."Private", "Indent"=1, "Can Read?"=TRUE, "Can Write?"=TRUE, "Is Read?"=FALSE, "Is Write?"=FALSE, "Inactive Parent?"=FALSE, "Unwired?"=FALSE}, {"Label"="Host Preferences Section", "Tag"="52.3.3a.Application:Host Preferences Section", "Property Type"=enum."Private", "Indent"=1, "Can Read?"=TRUE, "Can Write?"=FALSE, "Is Read?"=FALSE, "Is Write?"=FALSE, "Inactive Parent?"=FALSE, "Unwired?"=FALSE}, {"Label"="IgnoreUnresolvedDLLRef", "Tag"="53.3.113.Application:IgnoreUnresolvedDLLRef", "Property Type"=enum."Private", "Indent"=1, "Can Read?"=TRUE, "Can Write?"=FALSE, "Is Read?"=FALSE, "Is Write?"=FALSE, "Inactive Parent?"=FALSE, "Unwired?"=FALSE}, {"Label"="ImageTableCount", "Tag"="54.3.114.Application:ImageTableCount", "Property Type"=enum."Private", "Indent"=1, "Can Read?"=TRUE, "Can Write?"=FALSE, "Is Read?"=FALSE, "Is Write?"=FALSE, "Inactive Parent?"=FALSE, "Unwired?"=FALSE}, {"Label"="ImageTableMaxCount", "Tag"="55.3.110.Application:ImageTableMaxCount", "Property Type"=enum."Private", "Indent"=1, "Can Read?"=TRUE, "Can Write?"=FALSE, "Is Read?"=FALSE, "Is Write?"=FALSE, "Inactive Parent?"=FALSE, "Unwired?"=FALSE}, {"Label"="Installed Package", "Tag"="56.3.5f.Application:Installed Package", "Property Type"=enum."Private", "Indent"=1, "Can Read?"=TRUE, "Can Write?"=FALSE, "Is Read?"=FALSE, "Is Write?"=FALSE, "Inactive Parent?"=FALSE, "Unwired?"=FALSE}, {"Label"="InstCachePath", "Tag"="57.3.f5.Application:InstCachePath", "Property Type"=enum."Private", "Indent"=1, "Can Read?"=TRUE, "Can Write?"=FALSE, "Is Read?"=FALSE, "Is Write?"=FALSE, "Inactive Parent?"=FALSE, "Unwired?"=FALSE}, {"Label"="Internet Toolkit Installed", "Tag"="58.3.62.Application:Internet Toolkit Installed", "Property Type"=enum."Private", "Indent"=1, "Can Read?"=TRUE, "Can Write?"=TRUE, "Is Read?"=FALSE, "Is Write?"=FALSE, "Inactive Parent?"=FALSE, "Unwired?"=FALSE}, {"Label"="Is Build App Instance", "Tag"="59.3.da.Application:Is Build App Instance", "Property Type"=enum."Private", "Indent"=1, "Can Read?"=TRUE, "Can Write?"=TRUE, "Is Read?"=FALSE, "Is Write?"=FALSE, "Inactive Parent?"=FALSE, "Unwired?"=FALSE}, {"Label"="Is Compile Suppressed", "Tag"="60.3.f6.Application:Is Compile Suppressed", "Property Type"=enum."Private", "Indent"=1, "Can Read?"=TRUE, "Can Write?"=TRUE, "Is Read?"=FALSE, "Is Write?"=FALSE, "Inactive Parent?"=FALSE, "Unwired?"=FALSE}, {"Label"="Is Editor In MDI Mode", "Tag"="61.3.7d.Application:Is Editor In MDI Mode", "Property Type"=enum."Private", "Indent"=1, "Can Read?"=TRUE, "Can Write?"=FALSE, "Is Read?"=FALSE, "Is Write?"=FALSE, "Inactive Parent?"=FALSE, "Unwired?"=FALSE}, {"Label"="Is Migration Enabled", "Tag"="62.3.a6.Application:Is Migration Enabled", "Property Type"=enum."Private", "Indent"=1, "Can Read?"=TRUE, "Can Write?"=TRUE, "Is Read?"=FALSE, "Is Write?"=FALSE, "Inactive Parent?"=FALSE, "Unwired?"=FALSE}, {"Label"="Kind", "Tag"="63.1.3.Application:Kind", "Property Type"=enum."Base", "Indent"=1, "Can Read?"=TRUE, "Can Write?"=FALSE, "Is Read?"=FALSE, "Is Write?"=FALSE, "Inactive Parent?"=FALSE, "Unwired?"=FALSE}, {"Label"="Language", "Tag"="64.1.63.Application:Language", "Property Type"=enum."Base", "Indent"=1, "Can Read?"=TRUE, "Can Write?"=FALSE, "Is Read?"=FALSE, "Is Write?"=FALSE, "Inactive Parent?"=FALSE, "Unwired?"=FALSE}, {"Label"="Legacy Build App File Layout", "Tag"="65.3.dc.Application:Legacy Build App File Layout", "Property Type"=enum."Private", "Indent"=1, "Can Read?"=TRUE, "Can Write?"=FALSE, "Is Read?"=FALSE, "Is Write?"=FALSE, "Inactive Parent?"=FALSE, "Unwired?"=FALSE}, {"Label"="Let Private Context Run With XNode", "Tag"="66.3.aa.Application:Let Private Context Run With XNode", "Property Type"=enum."Private", "Indent"=1, "Can Read?"=TRUE, "Can Write?"=TRUE, "Is Read?"=FALSE, "Is Write?"=FALSE, "Inactive Parent?"=FALSE, "Unwired?"=FALSE}, {"Label"="Library Finish Partial Load Enabled", "Tag"="67.3.f9.Application:Library Finish Partial Load Enabled", "Property Type"=enum."Private", "Indent"=1, "Can Read?"=TRUE, "Can Write?"=TRUE, "Is Read?"=FALSE, "Is Write?"=FALSE, "Inactive Parent?"=FALSE, "Unwired?"=FALSE}, {"Label"="Lock Instantiations for AppBuilder", "Tag"="68.3.e3.Application:Lock Instantiations for AppBuilder", "Property Type"=enum."Private", "Indent"=1, "Can Read?"=TRUE, "Can Write?"=TRUE, "Is Read?"=FALSE, "Is Write?"=FALSE, "Inactive Parent?"=FALSE, "Unwired?"=FALSE}, {"Label"="Locked Down For Build", "Tag"="69.3.fd.Application:Locked Down For Build", "Property Type"=enum."Private", "Indent"=1, "Can Read?"=TRUE, "Can Write?"=TRUE, "Is Read?"=FALSE, "Is Write?"=FALSE, "Inactive Parent?"=FALSE, "Unwired?"=FALSE}, {"Label"="LVTarget", "Tag"="70.3.83.Application:LVTarget", "Property Type"=enum."Private", "Indent"=1, "Can Read?"=TRUE, "Can Write?"=FALSE, "Is Read?"=FALSE, "Is Write?"=FALSE, "Inactive Parent?"=FALSE, "Unwired?"=FALSE}, {"Label"="Mass Compile Warn On Read Only VIs", "Tag"="71.3.f4.Application:Mass Compile Warn On Read Only VIs", "Property Type"=enum."Private", "Indent"=1, "Can Read?"=TRUE, "Can Write?"=TRUE, "Is Read?"=FALSE, "Is Write?"=FALSE, "Inactive Parent?"=FALSE, "Unwired?"=FALSE}, {"Label"="Menu Launch", "Tag"="72.2.7f.Application:Menu Launch", "Property Type"=enum."Base", "Indent"=1, "Can Read?"=FALSE, "Can Write?"=FALSE, "Is Read?"=FALSE, "Is Write?"=FALSE, "Inactive Parent?"=TRUE, "Unwired?"=FALSE}, {"Label"="App", "Tag"="72.2.7f.Application:Menu Launch:App", "Property Type"=enum."Scripting", "Indent"=2, "Can Read?"=TRUE, "Can Write?"=FALSE, "Is Read?"=FALSE, "Is Write?"=FALSE, "Inactive Parent?"=FALSE, "Unwired?"=FALSE}, {"Label"="VI", "Tag"="73.2.1d.Application:Menu Launch:VI", "Property Type"=enum."Scripting", "Indent"=2, "Can Read?"=TRUE, "Can Write?"=FALSE, "Is Read?"=FALSE, "Is Write?"=FALSE, "Inactive Parent?"=FALSE, "Unwired?"=FALSE}, {"Label"="Multi Pwd Op Cancelled?", "Tag"="74.3.a4.Application:Multi Pwd Op Cancelled?", "Property Type"=enum."Private", "Indent"=1, "Can Read?"=TRUE, "Can Write?"=FALSE, "Is Read?"=FALSE, "Is Write?"=FALSE, "Inactive Parent?"=FALSE, "Unwired?"=FALSE}, {"Label"="Name", "Tag"="75.1.0.Application:Name", "Property Type"=enum."Base", "Indent"=1, "Can Read?"=TRUE, "Can Write?"=FALSE, "Is Read?"=FALSE, "Is Write?"=FALSE, "Inactive Parent?"=FALSE, "Unwired?"=FALSE}, {"Label"="NativeEventTracingEnabled", "Tag"="76.3.118.Application:NativeEventTracingEnabled", "Property Type"=enum."Private", "Indent"=1, "Can Read?"=TRUE, "Can Write?"=TRUE, "Is Read?"=FALSE, "Is Write?"=FALSE, "Inactive Parent?"=FALSE, "Unwired?"=FALSE}, {"Label"="On Line", "Tag"="77.3.97.Application:On Line", "Property Type"=enum."Private", "Indent"=1, "Can Read?"=TRUE, "Can Write?"=TRUE, "Is Read?"=FALSE, "Is Write?"=FALSE, "Inactive Parent?"=FALSE, "Unwired?"=FALSE}, {"Label"="Parent Window For Dialogs", "Tag"="78.3.36.Application:Parent Window For Dialogs", "Property Type"=enum."Private", "Indent"=1, "Can Read?"=TRUE, "Can Write?"=TRUE, "Is Read?"=FALSE, "Is Write?"=FALSE, "Inactive Parent?"=FALSE, "Unwired?"=FALSE}, {"Label"="PPL LoadInCompatible LVVersion Default Value", "Tag"="79.3.115.Application:PPL LoadInCompatible LVVersion Default Value", "Property Type"=enum."Private", "Indent"=1, "Can Read?"=TRUE, "Can Write?"=TRUE, "Is Read?"=FALSE, "Is Write?"=FALSE, "Inactive Parent?"=FALSE, "Unwired?"=FALSE}, {"Label"="Preferences File Path", "Tag"="80.3.39.Application:Preferences File Path", "Property Type"=enum."Private", "Indent"=1, "Can Read?"=TRUE, "Can Write?"=FALSE, "Is Read?"=FALSE, "Is Write?"=FALSE, "Inactive Parent?"=FALSE, "Unwired?"=FALSE}, {"Label"="Private?", "Tag"="81.3.84.Application:Private?", "Property Type"=enum."Private", "Indent"=1, "Can Read?"=TRUE, "Can Write?"=FALSE, "Is Read?"=FALSE, "Is Write?"=FALSE, "Inactive Parent?"=FALSE, "Unwired?"=FALSE}, {"Label"="Property and Method Data Types", "Tag"="82.3.be.Application:Property and Method Data Types", "Property Type"=enum."Private", "Indent"=1, "Can Read?"=TRUE, "Can Write?"=FALSE, "Is Read?"=FALSE, "Is Write?"=FALSE, "Inactive Parent?"=FALSE, "Unwired?"=FALSE}, {"Label"="Pump OS Messages", "Tag"="83.3.66.Application:Pump OS Messages", "Property Type"=enum."Private", "Indent"=1, "Can Read?"=TRUE, "Can Write?"=TRUE, "Is Read?"=FALSE, "Is Write?"=FALSE, "Inactive Parent?"=FALSE, "Unwired?"=FALSE}, {"Label"="Real-Time Support", "Tag"="84.3.59.Application:Real-Time Support", "Property Type"=enum."Private", "Indent"=1, "Can Read?"=TRUE, "Can Write?"=FALSE, "Is Read?"=FALSE, "Is Write?"=FALSE, "Inactive Parent?"=FALSE, "Unwired?"=FALSE}, {"Label"="Registered Organization", "Tag"="85.3.3c.Application:Registered Organization", "Property Type"=enum."Private", "Indent"=1, "Can Read?"=TRUE, "Can Write?"=FALSE, "Is Read?"=FALSE, "Is Write?"=FALSE, "Inactive Parent?"=FALSE, "Unwired?"=FALSE}, {"Label"="Registered Owner", "Tag"="86.3.3b.Application:Registered Owner", "Property Type"=enum."Private", "Indent"=1, "Can Read?"=TRUE, "Can Write?"=FALSE, "Is Read?"=FALSE, "Is Write?"=FALSE, "Inactive Parent?"=FALSE, "Unwired?"=FALSE}, {"Label"="Remote Web Server Active", "Tag"="87.3.45.Application:Remote Web Server Active", "Property Type"=enum."Private", "Indent"=1, "Can Read?"=TRUE, "Can Write?"=FALSE, "Is Read?"=FALSE, "Is Write?"=FALSE, "Inactive Parent?"=FALSE, "Unwired?"=FALSE}, {"Label"="Rename Variables for AppBuilder", "Tag"="88.3.ed.Application:Rename Variables for AppBuilder", "Property Type"=enum."Private", "Indent"=1, "Can Read?"=TRUE, "Can Write?"=TRUE, "Is Read?"=FALSE, "Is Write?"=FALSE, "Inactive Parent?"=FALSE, "Unwired?"=FALSE}, {"Label"="Save Format", "Tag"="89.3.89.Application:Save Format", "Property Type"=enum."Private", "Indent"=1, "Can Read?"=TRUE, "Can Write?"=TRUE, "Is Read?"=FALSE, "Is Write?"=FALSE, "Inactive Parent?"=FALSE, "Unwired?"=FALSE}, {"Label"="Save Version", "Tag"="90.1.de.Application:Save Version", "Property Type"=enum."Base", "Indent"=1, "Can Read?"=TRUE, "Can Write?"=FALSE, "Is Read?"=FALSE, "Is Write?"=FALSE, "Inactive Parent?"=FALSE, "Unwired?"=FALSE}, {"Label"="Save Version As Integer", "Tag"="91.3.df.Application:Save Version As Integer", "Property Type"=enum."Private", "Indent"=1, "Can Read?"=TRUE, "Can Write?"=FALSE, "Is Read?"=FALSE, "Is Write?"=FALSE, "Inactive Parent?"=FALSE, "Unwired?"=FALSE}, {"Label"="Saveable Versions", "Tag"="92.1.b9.Application:Saveable Versions", "Property Type"=enum."Base", "Indent"=1, "Can Read?"=TRUE, "Can Write?"=FALSE, "Is Read?"=FALSE, "Is Write?"=FALSE, "Inactive Parent?"=FALSE, "Unwired?"=FALSE}, {"Label"="SaveChangesAutoSelection", "Tag"="93.3.117.Application:SaveChangesAutoSelection", "Property Type"=enum."Private", "Indent"=1, "Can Read?"=TRUE, "Can Write?"=TRUE, "Is Read?"=FALSE, "Is Write?"=FALSE, "Inactive Parent?"=FALSE, "Unwired?"=FALSE}, {"Label"="Search Paths", "Tag"="94.3.58.Application:Search Paths", "Property Type"=enum."Private", "Indent"=1, "Can Read?"=TRUE, "Can Write?"=TRUE, "Is Read?"=FALSE, "Is Write?"=FALSE, "Inactive Parent?"=FALSE, "Unwired?"=FALSE}, {"Label"="Selection List Changed", "Tag"="95.3.47.Application:Selection List Changed", "Property Type"=enum."Private", "Indent"=1, "Can Read?"=TRUE, "Can Write?"=FALSE, "Is Read?"=FALSE, "Is Write?"=FALSE, "Inactive Parent?"=FALSE, "Unwired?"=FALSE}, {"Label"="Selective Deallocation", "Tag"="96.3.103.Application:Selective Deallocation", "Property Type"=enum."Private", "Indent"=1, "Can Read?"=TRUE, "Can Write?"=TRUE, "Is Read?"=FALSE, "Is Write?"=FALSE, "Inactive Parent?"=FALSE, "Unwired?"=FALSE}, {"Label"="EnableForAllVIs", "Tag"="97.3.104.Application:Selective Deallocation:EnableForAllVIs", "Property Type"=enum."Private", "Indent"=2, "Can Read?"=TRUE, "Can Write?"=TRUE, "Is Read?"=FALSE, "Is Write?"=FALSE, "Inactive Parent?"=FALSE, "Unwired?"=FALSE}, {"Label"="LargeBufferThreshold", "Tag"="98.3.105.Application:Selective Deallocation:LargeBufferThreshold", "Property Type"=enum."Private", "Indent"=2, "Can Read?"=TRUE, "Can Write?"=TRUE, "Is Read?"=FALSE, "Is Write?"=FALSE, "Inactive Parent?"=FALSE, "Unwired?"=FALSE}, {"Label"="Serial Number", "Tag"="99.3.3d.Application:Serial Number", "Property Type"=enum."Private", "Indent"=1, "Can Read?"=TRUE, "Can Write?"=FALSE, "Is Read?"=FALSE, "Is Write?"=FALSE, "Inactive Parent?"=FALSE, "Unwired?"=FALSE}, {"Label"="Show FP Tip Strips", "Tag"="100.1.3f.Application:Show FP Tip Strips", "Property Type"=enum."Base", "Indent"=1, "Can Read?"=TRUE, "Can Write?"=TRUE, "Is Read?"=FALSE, "Is Write?"=FALSE, "Inactive Parent?"=FALSE, "Unwired?"=FALSE}, {"Label"="ShowAutoErrDialog", "Tag"="101.3.102.Application:ShowAutoErrDialog", "Property Type"=enum."Private", "Indent"=1, "Can Read?"=TRUE, "Can Write?"=TRUE, "Is Read?"=FALSE, "Is Write?"=FALSE, "Inactive Parent?"=FALSE, "Unwired?"=FALSE}, {"Label"="Target", "Tag"="102.3.8b.Application:Target", "Property Type"=enum."Base", "Indent"=1, "Can Read?"=FALSE, "Can Write?"=FALSE, "Is Read?"=FALSE, "Is Write?"=FALSE, "Inactive Parent?"=TRUE, "Unwired?"=FALSE}, {"Label"="Class Name", "Tag"="102.3.8b.Application:Target:Class Name", "Property Type"=enum."Private", "Indent"=2, "Can Read?"=TRUE, "Can Write?"=FALSE, "Is Read?"=FALSE, "Is Write?"=FALSE, "Inactive Parent?"=FALSE, "Unwired?"=FALSE}, {"Label"="CPU", "Tag"="103.1.5.Application:Target:CPU", "Property Type"=enum."Base", "Indent"=2, "Can Read?"=TRUE, "Can Write?"=FALSE, "Is Read?"=FALSE, "Is Write?"=FALSE, "Inactive Parent?"=FALSE, "Unwired?"=FALSE}, {"Label"="Current Processor ID", "Tag"="104.3.d2.Application:Target:Current Processor ID", "Property Type"=enum."Private", "Indent"=2, "Can Read?"=TRUE, "Can Write?"=FALSE, "Is Read?"=FALSE, "Is Write?"=FALSE, "Inactive Parent?"=FALSE, "Unwired?"=FALSE}, {"Label"="Data Cache Entry Sizes", "Tag"="105.1.d3.Application:Target:Data Cache Entry Sizes", "Property Type"=enum."Base", "Indent"=2, "Can Read?"=TRUE, "Can Write?"=FALSE, "Is Read?"=FALSE, "Is Write?"=FALSE, "Inactive Parent?"=FALSE, "Unwired?"=FALSE}, {"Label"="Data Cache Sizes", "Tag"="106.1.d4.Application:Target:Data Cache Sizes", "Property Type"=enum."Base", "Indent"=2, "Can Read?"=TRUE, "Can Write?"=FALSE, "Is Read?"=FALSE, "Is Write?"=FALSE, "Inactive Parent?"=FALSE, "Unwired?"=FALSE}, {"Label"="Info", "Tag"="107.3.54.Application:Target:Info", "Property Type"=enum."Private", "Indent"=2, "Can Read?"=TRUE, "Can Write?"=FALSE, "Is Read?"=FALSE, "Is Write?"=FALSE, "Inactive Parent?"=FALSE, "Unwired?"=FALSE}, {"Label"="IP Address", "Tag"="108.3.44.Application:Target:IP Address", "Property Type"=enum."Private", "Indent"=2, "Can Read?"=TRUE, "Can Write?"=FALSE, "Is Read?"=FALSE, "Is Write?"=FALSE, "Inactive Parent?"=FALSE, "Unwired?"=FALSE}, {"Label"="Number of Cores per Package", "Tag"="109.1.d0.Application:Target:Number of Cores per Package", "Property Type"=enum."Base", "Indent"=2, "Can Read?"=TRUE, "Can Write?"=FALSE, "Is Read?"=FALSE, "Is Write?"=FALSE, "Inactive Parent?"=FALSE, "Unwired?"=FALSE}, {"Label"="Number of Logical Processors", "Tag"="110.1.ce.Application:Target:Number of Logical Processors", "Property Type"=enum."Base", "Indent"=2, "Can Read?"=TRUE, "Can Write?"=FALSE, "Is Read?"=FALSE, "Is Write?"=FALSE, "Inactive Parent?"=FALSE, "Unwired?"=FALSE}, {"Label"="Number of Logical Processors per Core", "Tag"="111.1.d1.Application:Target:Number of Logical Processors per Core", "Property Type"=enum."Base", "Indent"=2, "Can Read?"=TRUE, "Can Write?"=FALSE, "Is Read?"=FALSE, "Is Write?"=FALSE, "Inactive Parent?"=FALSE, "Unwired?"=FALSE}, {"Label"="Number of Packages", "Tag"="112.1.d5.Application:Target:Number of Packages", "Property Type"=enum."Base", "Indent"=2, "Can Read?"=TRUE, "Can Write?"=FALSE, "Is Read?"=FALSE, "Is Write?"=FALSE, "Inactive Parent?"=FALSE, "Unwired?"=FALSE}, {"Label"="Operating System", "Tag"="113.1.4.Application:Target:Operating System", "Property Type"=enum."Base", "Indent"=2, "Can Read?"=TRUE, "Can Write?"=FALSE, "Is Read?"=FALSE, "Is Write?"=FALSE, "Inactive Parent?"=FALSE, "Unwired?"=FALSE}, {"Label"="TestStandOptions", "Tag"="114.3.db.Application:TestStandOptions", "Property Type"=enum."Private", "Indent"=1, "Can Read?"=TRUE, "Can Write?"=TRUE, "Is Read?"=FALSE, "Is Write?"=FALSE, "Inactive Parent?"=FALSE, "Unwired?"=FALSE}, {"Label"="Tools Palette Open", "Tag"="115.3.2c.Application:Tools Palette Open", "Property Type"=enum."Private", "Indent"=1, "Can Read?"=TRUE, "Can Write?"=TRUE, "Is Read?"=FALSE, "Is Write?"=FALSE, "Inactive Parent?"=FALSE, "Unwired?"=FALSE}, {"Label"="Treat LV 2016 As Binary Compatible", "Tag"="116.3.116.Application:Treat LV 2016 As Binary Compatible", "Property Type"=enum."Private", "Indent"=1, "Can Read?"=TRUE, "Can Write?"=TRUE, "Is Read?"=FALSE, "Is Write?"=FALSE, "Inactive Parent?"=FALSE, "Unwired?"=FALSE}, {"Label"="UD Refnum Files", "Tag"="117.3.ec.Application:UD Refnum Files", "Property Type"=enum."Private", "Indent"=1, "Can Read?"=TRUE, "Can Write?"=FALSE, "Is Read?"=FALSE, "Is Write?"=FALSE, "Inactive Parent?"=FALSE, "Unwired?"=FALSE}, {"Label"="Unattended Mode", "Tag"="118.3.4d.Application:Unattended Mode", "Property Type"=enum."Private", "Indent"=1, "Can Read?"=TRUE, "Can Write?"=TRUE, "Is Read?"=FALSE, "Is Write?"=FALSE, "Inactive Parent?"=FALSE, "Unwired?"=FALSE}, {"Label"="Use App Template Browser", "Tag"="119.3.51.Application:Use App Template Browser", "Property Type"=enum."Private", "Indent"=1, "Can Read?"=TRUE, "Can Write?"=TRUE, "Is Read?"=FALSE, "Is Write?"=FALSE, "Inactive Parent?"=FALSE, "Unwired?"=FALSE}, {"Label"="User Interface Available", "Tag"="120.1.5a.Application:User Interface Available", "Property Type"=enum."Base", "Indent"=1, "Can Read?"=TRUE, "Can Write?"=FALSE, "Is Read?"=FALSE, "Is Write?"=FALSE, "Inactive Parent?"=FALSE, "Unwired?"=FALSE}, {"Label"="User Name", "Tag"="121.1.1.Application:User Name", "Property Type"=enum."Base", "Indent"=1, "Can Read?"=TRUE, "Can Write?"=TRUE, "Is Read?"=FALSE, "Is Write?"=FALSE, "Inactive Parent?"=FALSE, "Unwired?"=FALSE}, {"Label"="Version As Integer", "Tag"="122.3.37.Application:Version As Integer", "Property Type"=enum."Private", "Indent"=1, "Can Read?"=TRUE, "Can Write?"=FALSE, "Is Read?"=FALSE, "Is Write?"=FALSE, "Inactive Parent?"=FALSE, "Unwired?"=FALSE}, {"Label"="Version Number", "Tag"="123.1.2.Application:Version Number", "Property Type"=enum."Base", "Indent"=1, "Can Read?"=TRUE, "Can Write?"=FALSE, "Is Read?"=FALSE, "Is Write?"=FALSE, "Inactive Parent?"=FALSE, "Unwired?"=FALSE}, {"Label"="Version Year", "Tag"="124.1.d7.Application:Version Year", "Property Type"=enum."Base", "Indent"=1, "Can Read?"=TRUE, "Can Write?"=FALSE, "Is Read?"=FALSE, "Is Write?"=FALSE, "Inactive Parent?"=FALSE, "Unwired?"=FALSE}, {"Label"="Version Year Number Only", "Tag"="125.3.109.Application:Version Year Number Only", "Property Type"=enum."Private", "Indent"=1, "Can Read?"=TRUE, "Can Write?"=FALSE, "Is Read?"=FALSE, "Is Write?"=FALSE, "Inactive Parent?"=FALSE, "Unwired?"=FALSE}, {"Label"="VI Of Top Most Block Diagram", "Tag"="126.2.9e.Application:VI Of Top Most Block Diagram", "Property Type"=enum."Scripting", "Indent"=1, "Can Read?"=TRUE, "Can Write?"=FALSE, "Is Read?"=FALSE, "Is Write?"=FALSE, "Inactive Parent?"=FALSE, "Unwired?"=FALSE}, {"Label"="Window For Panel Origin", "Tag"="127.3.64.Application:Window For Panel Origin", "Property Type"=enum."Private", "Indent"=1, "Can Read?"=TRUE, "Can Write?"=TRUE, "Is Read?"=FALSE, "Is Write?"=FALSE, "Inactive Parent?"=FALSE, "Unwired?"=FALSE}, {"Label"="Z Compress Level", "Tag"="128.3.96.Application:Z Compress Level", "Property Type"=enum."Private", "Indent"=1, "Can Read?"=TRUE, "Can Write?"=TRUE, "Is Read?"=FALSE, "Is Write?"=FALSE, "Inactive Parent?"=FALSE, "Unwired?"=FALSE}, {"Label"="Crosslink", "Tag"="129.3.a7.Crosslink", "Property Type"=enum."Base", "Indent"=0, "Can Read?"=FALSE, "Can Write?"=FALSE, "Is Read?"=FALSE, "Is Write?"=FALSE, "Inactive Parent?"=TRUE, "Unwired?"=FALSE}, {"Label"="Force Enable Dialogs", "Tag"="129.3.a7.Crosslink:Force Enable Dialogs", "Property Type"=enum."Private", "Indent"=1, "Can Read?"=TRUE, "Can Write?"=TRUE, "Is Read?"=FALSE, "Is Write?"=FALSE, "Inactive Parent?"=FALSE, "Unwired?"=FALSE}, {"Label"="Suppress Dialogs", "Tag"="130.3.a8.Crosslink:Suppress Dialogs", "Property Type"=enum."Private", "Indent"=1, "Can Read?"=TRUE, "Can Write?"=TRUE, "Is Read?"=FALSE, "Is Write?"=FALSE, "Inactive Parent?"=FALSE, "Unwired?"=FALSE}, {"Label"="Debug Server", "Tag"="131.1.98.Debug Server", "Property Type"=enum."Base", "Indent"=0, "Can Read?"=FALSE, "Can Write?"=FALSE, "Is Read?"=FALSE, "Is Write?"=FALSE, "Inactive Parent?"=TRUE, "Unwired?"=FALSE}, {"Label"="Server Active", "Tag"="131.1.98.Debug Server:Server Active", "Property Type"=enum."Base", "Indent"=1, "Can Read?"=TRUE, "Can Write?"=TRUE, "Is Read?"=FALSE, "Is Write?"=FALSE, "Inactive Parent?"=FALSE, "Unwired?"=FALSE}, {"Label"="TCP/IP Access List", "Tag"="132.1.99.Debug Server:TCP/IP Access List", "Property Type"=enum."Base", "Indent"=1, "Can Read?"=TRUE, "Can Write?"=TRUE, "Is Read?"=FALSE, "Is Write?"=FALSE, "Inactive Parent?"=FALSE, "Unwired?"=FALSE}, {"Label"="Delay File Notifications", "Tag"="133.3.a2.Delay File Notifications", "Property Type"=enum."Private", "Indent"=0, "Can Read?"=TRUE, "Can Write?"=TRUE, "Is Read?"=FALSE, "Is Write?"=FALSE, "Inactive Parent?"=FALSE, "Unwired?"=FALSE}, {"Label"="Display", "Tag"="134.1.22.Display", "Property Type"=enum."Base", "Indent"=0, "Can Read?"=FALSE, "Can Write?"=FALSE, "Is Read?"=FALSE, "Is Write?"=FALSE, "Inactive Parent?"=TRUE, "Unwired?"=FALSE}, {"Label"="All Monitors", "Tag"="134.1.22.Display:All Monitors", "Property Type"=enum."Base", "Indent"=1, "Can Read?"=TRUE, "Can Write?"=FALSE, "Is Read?"=FALSE, "Is Write?"=FALSE, "Inactive Parent?"=FALSE, "Unwired?"=FALSE}, {"Label"="Primary Workspace", "Tag"="135.1.21.Display:Primary Workspace", "Property Type"=enum."Base", "Indent"=1, "Can Read?"=TRUE, "Can Write?"=FALSE, "Is Read?"=FALSE, "Is Write?"=FALSE, "Inactive Parent?"=FALSE, "Unwired?"=FALSE}, {"Label"="Get NXT Context", "Tag"="136.3.e0.Get NXT Context", "Property Type"=enum."Private", "Indent"=0, "Can Read?"=TRUE, "Can Write?"=FALSE, "Is Read?"=FALSE, "Is Write?"=FALSE, "Inactive Parent?"=FALSE, "Unwired?"=FALSE}, {"Label"="Load and Save Warnings", "Tag"="137.3.bb.Load and Save Warnings", "Property Type"=enum."Base", "Indent"=0, "Can Read?"=FALSE, "Can Write?"=FALSE, "Is Read?"=FALSE, "Is Write?"=FALSE, "Inactive Parent?"=TRUE, "Unwired?"=FALSE}, {"Label"="Auto Test Mode", "Tag"="137.3.bb.Load and Save Warnings:Auto Test Mode", "Property Type"=enum."Private", "Indent"=1, "Can Read?"=TRUE, "Can Write?"=TRUE, "Is Read?"=FALSE, "Is Write?"=FALSE, "Inactive Parent?"=FALSE, "Unwired?"=FALSE}, {"Label"="History", "Tag"="138.3.bc.Load and Save Warnings:History", "Property Type"=enum."Private", "Indent"=1, "Can Read?"=TRUE, "Can Write?"=FALSE, "Is Read?"=FALSE, "Is Write?"=FALSE, "Inactive Parent?"=FALSE, "Unwired?"=FALSE}, {"Label"="MathScript", "Tag"="139.3.a5.MathScript", "Property Type"=enum."Base", "Indent"=0, "Can Read?"=FALSE, "Can Write?"=FALSE, "Is Read?"=FALSE, "Is Write?"=FALSE, "Inactive Parent?"=TRUE, "Unwired?"=FALSE}, {"Label"="All M Files In Context", "Tag"="139.3.a5.MathScript:All M Files In Context", "Property Type"=enum."Private", "Indent"=1, "Can Read?"=TRUE, "Can Write?"=FALSE, "Is Read?"=FALSE, "Is Write?"=FALSE, "Inactive Parent?"=FALSE, "Unwired?"=FALSE}, {"Label"="ColorsInSync", "Tag"="140.3.f1.MathScript:ColorsInSync", "Property Type"=enum."Private", "Indent"=1, "Can Read?"=TRUE, "Can Write?"=TRUE, "Is Read?"=FALSE, "Is Write?"=FALSE, "Inactive Parent?"=FALSE, "Unwired?"=FALSE}, {"Label"="Compiler Signature", "Tag"="141.3.e8.MathScript:Compiler Signature", "Property Type"=enum."Private", "Indent"=1, "Can Read?"=TRUE, "Can Write?"=FALSE, "Is Read?"=FALSE, "Is Write?"=FALSE, "Inactive Parent?"=FALSE, "Unwired?"=FALSE}, {"Label"="CompilerInMemory", "Tag"="142.3.f2.MathScript:CompilerInMemory", "Property Type"=enum."Private", "Indent"=1, "Can Read?"=TRUE, "Can Write?"=FALSE, "Is Read?"=FALSE, "Is Write?"=FALSE, "Inactive Parent?"=FALSE, "Unwired?"=FALSE}, {"Label"="HighlightingColors", "Tag"="143.3.f0.MathScript:HighlightingColors", "Property Type"=enum."Private", "Indent"=1, "Can Read?"=TRUE, "Can Write?"=FALSE, "Is Read?"=FALSE, "Is Write?"=FALSE, "Inactive Parent?"=FALSE, "Unwired?"=FALSE}, {"Label"="Path", "Tag"="144.3.a3.MathScript:Path", "Property Type"=enum."Private", "Indent"=1, "Can Read?"=TRUE, "Can Write?"=FALSE, "Is Read?"=FALSE, "Is Write?"=FALSE, "Inactive Parent?"=FALSE, "Unwired?"=FALSE}, {"Label"="Module Handle", "Tag"="145.3.65.Module Handle", "Property Type"=enum."Private", "Indent"=0, "Can Read?"=TRUE, "Can Write?"=FALSE, "Is Read?"=FALSE, "Is Write?"=FALSE, "Inactive Parent?"=FALSE, "Unwired?"=FALSE}, {"Label"="NI Security", "Tag"="146.1.a0.NI Security", "Property Type"=enum."Base", "Indent"=0, "Can Read?"=FALSE, "Can Write?"=FALSE, "Is Read?"=FALSE, "Is Write?"=FALSE, "Inactive Parent?"=TRUE, "Unwired?"=FALSE}, {"Label"="Nobody Logged In?", "Tag"="146.1.a0.NI Security:Nobody Logged In?", "Property Type"=enum."Base", "Indent"=1, "Can Read?"=TRUE, "Can Write?"=FALSE, "Is Read?"=FALSE, "Is Write?"=FALSE, "Inactive Parent?"=FALSE, "Unwired?"=FALSE}, {"Label"="Unique User", "Tag"="147.3.a1.NI Security:Unique User", "Property Type"=enum."Private", "Indent"=1, "Can Read?"=TRUE, "Can Write?"=FALSE, "Is Read?"=FALSE, "Is Write?"=FALSE, "Inactive Parent?"=FALSE, "Unwired?"=FALSE}, {"Label"="User", "Tag"="148.1.7c.NI Security:User", "Property Type"=enum."Base", "Indent"=1, "Can Read?"=TRUE, "Can Write?"=FALSE, "Is Read?"=FALSE, "Is Write?"=FALSE, "Inactive Parent?"=FALSE, "Unwired?"=FALSE}, {"Label"="Operating System", "Tag"="149.1.bf.Operating System", "Property Type"=enum."Base", "Indent"=0, "Can Read?"=FALSE, "Can Write?"=FALSE, "Is Read?"=FALSE, "Is Write?"=FALSE, "Inactive Parent?"=TRUE, "Unwired?"=FALSE}, {"Label"="Build Number", "Tag"="149.1.bf.Operating System:Build Number", "Property Type"=enum."Base", "Indent"=1, "Can Read?"=TRUE, "Can Write?"=FALSE, "Is Read?"=FALSE, "Is Write?"=FALSE, "Inactive Parent?"=FALSE, "Unwired?"=FALSE}, {"Label"="Detailed Name", "Tag"="150.1.c6.Operating System:Detailed Name", "Property Type"=enum."Base", "Indent"=1, "Can Read?"=TRUE, "Can Write?"=FALSE, "Is Read?"=FALSE, "Is Write?"=FALSE, "Inactive Parent?"=FALSE, "Unwired?"=FALSE}, {"Label"="Name", "Tag"="151.1.6.Operating System:Name", "Property Type"=enum."Base", "Indent"=1, "Can Read?"=TRUE, "Can Write?"=FALSE, "Is Read?"=FALSE, "Is Write?"=FALSE, "Inactive Parent?"=FALSE, "Unwired?"=FALSE}, {"Label"="Version Number", "Tag"="152.1.7.Operating System:Version Number", "Property Type"=enum."Base", "Indent"=1, "Can Read?"=TRUE, "Can Write?"=FALSE, "Is Read?"=FALSE, "Is Write?"=FALSE, "Inactive Parent?"=FALSE, "Unwired?"=FALSE}, {"Label"="Options", "Tag"="153.3.8c.Options", "Property Type"=enum."Base", "Indent"=0, "Can Read?"=FALSE, "Can Write?"=FALSE, "Is Read?"=FALSE, "Is Write?"=FALSE, "Inactive Parent?"=TRUE, "Unwired?"=FALSE}, {"Label"="Editor Menu Bar", "Tag"="153.3.8c.Options:Editor Menu Bar", "Property Type"=enum."Private", "Indent"=1, "Can Read?"=TRUE, "Can Write?"=FALSE, "Is Read?"=FALSE, "Is Write?"=FALSE, "Inactive Parent?"=FALSE, "Unwired?"=FALSE}, {"Label"="Use Abridged Menus", "Tag"="154.3.6b.Options:Use Abridged Menus", "Property Type"=enum."Private", "Indent"=1, "Can Read?"=TRUE, "Can Write?"=TRUE, "Is Read?"=FALSE, "Is Write?"=FALSE, "Inactive Parent?"=FALSE, "Unwired?"=FALSE}, {"Label"="Palettes", "Tag"="155.3.b2.Palettes", "Property Type"=enum."Base", "Indent"=0, "Can Read?"=FALSE, "Can Write?"=FALSE, "Is Read?"=FALSE, "Is Write?"=FALSE, "Inactive Parent?"=TRUE, "Unwired?"=FALSE}, {"Label"="Get Controls Names", "Tag"="155.3.b2.Palettes:Get Controls Names", "Property Type"=enum."Private", "Indent"=1, "Can Read?"=TRUE, "Can Write?"=FALSE, "Is Read?"=FALSE, "Is Write?"=FALSE, "Inactive Parent?"=FALSE, "Unwired?"=FALSE}, {"Label"="Get Functions Names", "Tag"="156.3.b1.Palettes:Get Functions Names", "Property Type"=enum."Private", "Indent"=1, "Can Read?"=TRUE, "Can Write?"=FALSE, "Is Read?"=FALSE, "Is Write?"=FALSE, "Inactive Parent?"=FALSE, "Unwired?"=FALSE}, {"Label"="Printing", "Tag"="157.1.4b.Printing", "Property Type"=enum."Base", "Indent"=0, "Can Read?"=FALSE, "Can Write?"=FALSE, "Is Read?"=FALSE, "Is Write?"=FALSE, "Inactive Parent?"=TRUE, "Unwired?"=FALSE}, {"Label"="Available Printers", "Tag"="157.1.4b.Printing:Available Printers", "Property Type"=enum."Base", "Indent"=1, "Can Read?"=TRUE, "Can Write?"=FALSE, "Is Read?"=FALSE, "Is Write?"=FALSE, "Inactive Parent?"=FALSE, "Unwired?"=FALSE}, {"Label"="Color/Grayscale?", "Tag"="158.1.48.Printing:Color/Grayscale?", "Property Type"=enum."Base", "Indent"=1, "Can Read?"=TRUE, "Can Write?"=TRUE, "Is Read?"=FALSE, "Is Write?"=FALSE, "Inactive Parent?"=FALSE, "Unwired?"=FALSE}, {"Label"="Custom All Controls?", "Tag"="159.1.29.Printing:Custom All Controls?", "Property Type"=enum."Base", "Indent"=1, "Can Read?"=TRUE, "Can Write?"=TRUE, "Is Read?"=FALSE, "Is Write?"=FALSE, "Inactive Parent?"=FALSE, "Unwired?"=FALSE}, {"Label"="Custom Cluster Constants?", "Tag"="160.1.e7.Printing:Custom Cluster Constants?", "Property Type"=enum."Base", "Indent"=1, "Can Read?"=TRUE, "Can Write?"=TRUE, "Is Read?"=FALSE, "Is Write?"=FALSE, "Inactive Parent?"=FALSE, "Unwired?"=FALSE}, {"Label"="Custom Connector?", "Tag"="161.1.c.Printing:Custom Connector?", "Property Type"=enum."Base", "Indent"=1, "Can Read?"=TRUE, "Can Write?"=TRUE, "Is Read?"=FALSE, "Is Write?"=FALSE, "Inactive Parent?"=FALSE, "Unwired?"=FALSE}, {"Label"="Custom Control Descriptions?", "Tag"="162.1.11.Printing:Custom Control Descriptions?", "Property Type"=enum."Base", "Indent"=1, "Can Read?"=TRUE, "Can Write?"=TRUE, "Is Read?"=FALSE, "Is Write?"=FALSE, "Inactive Parent?"=FALSE, "Unwired?"=FALSE}, {"Label"="Custom Control Label/Caption?", "Tag"="163.1.93.Printing:Custom Control Label/Caption?", "Property Type"=enum."Base", "Indent"=1, "Can Read?"=TRUE, "Can Write?"=TRUE, "Is Read?"=FALSE, "Is Write?"=FALSE, "Inactive Parent?"=FALSE, "Unwired?"=FALSE}, {"Label"="Custom Control Types?", "Tag"="164.1.12.Printing:Custom Control Types?", "Property Type"=enum."Base", "Indent"=1, "Can Read?"=TRUE, "Can Write?"=TRUE, "Is Read?"=FALSE, "Is Write?"=FALSE, "Inactive Parent?"=FALSE, "Unwired?"=FALSE}, {"Label"="Custom Controls?", "Tag"="165.1.10.Printing:Custom Controls?", "Property Type"=enum."Base", "Indent"=1, "Can Read?"=TRUE, "Can Write?"=TRUE, "Is Read?"=FALSE, "Is Write?"=FALSE, "Inactive Parent?"=FALSE, "Unwired?"=FALSE}, {"Label"="Custom Description?", "Tag"="166.1.d.Printing:Custom Description?", "Property Type"=enum."Base", "Indent"=1, "Can Read?"=TRUE, "Can Write?"=TRUE, "Is Read?"=FALSE, "Is Write?"=FALSE, "Inactive Parent?"=FALSE, "Unwired?"=FALSE}, {"Label"="Custom Diagram Hidden?", "Tag"="167.1.14.Printing:Custom Diagram Hidden?", "Property Type"=enum."Base", "Indent"=1, "Can Read?"=TRUE, "Can Write?"=TRUE, "Is Read?"=FALSE, "Is Write?"=FALSE, "Inactive Parent?"=FALSE, "Unwired?"=FALSE}, {"Label"="Custom Diagram Repeat?", "Tag"="168.1.15.Printing:Custom Diagram Repeat?", "Property Type"=enum."Base", "Indent"=1, "Can Read?"=TRUE, "Can Write?"=TRUE, "Is Read?"=FALSE, "Is Write?"=FALSE, "Inactive Parent?"=FALSE, "Unwired?"=FALSE}, {"Label"="Custom Diagram?", "Tag"="169.1.13.Printing:Custom Diagram?", "Property Type"=enum."Base", "Indent"=1, "Can Read?"=TRUE, "Can Write?"=TRUE, "Is Read?"=FALSE, "Is Write?"=FALSE, "Inactive Parent?"=FALSE, "Unwired?"=FALSE}, {"Label"="Custom Express VI Configuration?", "Tag"="170.1.5c.Printing:Custom Express VI Configuration?", "Property Type"=enum."Base", "Indent"=1, "Can Read?"=TRUE, "Can Write?"=TRUE, "Is Read?"=FALSE, "Is Write?"=FALSE, "Inactive Parent?"=FALSE, "Unwired?"=FALSE}, {"Label"="Custom Hierarchy?", "Tag"="171.1.17.Printing:Custom Hierarchy?", "Property Type"=enum."Base", "Indent"=1, "Can Read?"=TRUE, "Can Write?"=TRUE, "Is Read?"=FALSE, "Is Write?"=FALSE, "Inactive Parent?"=FALSE, "Unwired?"=FALSE}, {"Label"="Custom History?", "Tag"="172.1.18.Printing:Custom History?", "Property Type"=enum."Base", "Indent"=1, "Can Read?"=TRUE, "Can Write?"=TRUE, "Is Read?"=FALSE, "Is Write?"=FALSE, "Inactive Parent?"=FALSE, "Unwired?"=FALSE}, {"Label"="Custom List of SubVIs?", "Tag"="173.1.16.Printing:Custom List of SubVIs?", "Property Type"=enum."Base", "Indent"=1, "Can Read?"=TRUE, "Can Write?"=TRUE, "Is Read?"=FALSE, "Is Write?"=FALSE, "Inactive Parent?"=FALSE, "Unwired?"=FALSE}, {"Label"="Custom Panel Border?", "Tag"="174.1.f.Printing:Custom Panel Border?", "Property Type"=enum."Base", "Indent"=1, "Can Read?"=TRUE, "Can Write?"=TRUE, "Is Read?"=FALSE, "Is Write?"=FALSE, "Inactive Parent?"=FALSE, "Unwired?"=FALSE}, {"Label"="Custom Panel?", "Tag"="175.1.e.Printing:Custom Panel?", "Property Type"=enum."Base", "Indent"=1, "Can Read?"=TRUE, "Can Write?"=TRUE, "Is Read?"=FALSE, "Is Write?"=FALSE, "Inactive Parent?"=FALSE, "Unwired?"=FALSE}, {"Label"="Default Printer", "Tag"="176.1.49.Printing:Default Printer", "Property Type"=enum."Base", "Indent"=1, "Can Read?"=TRUE, "Can Write?"=TRUE, "Is Read?"=FALSE, "Is Write?"=FALSE, "Inactive Parent?"=FALSE, "Unwired?"=FALSE}, {"Label"="File Wrap Text Length", "Tag"="177.1.9.Printing:File Wrap Text Length", "Property Type"=enum."Base", "Indent"=1, "Can Read?"=TRUE, "Can Write?"=TRUE, "Is Read?"=FALSE, "Is Write?"=FALSE, "Inactive Parent?"=FALSE, "Unwired?"=FALSE}, {"Label"="JPEG Quality", "Tag"="178.1.b.Printing:JPEG Quality", "Property Type"=enum."Base", "Indent"=1, "Can Read?"=TRUE, "Can Write?"=TRUE, "Is Read?"=FALSE, "Is Write?"=FALSE, "Inactive Parent?"=FALSE, "Unwired?"=FALSE}, {"Label"="Method", "Tag"="179.1.4a.Printing:Method", "Property Type"=enum."Base", "Indent"=1, "Can Read?"=TRUE, "Can Write?"=TRUE, "Is Read?"=FALSE, "Is Write?"=FALSE, "Inactive Parent?"=FALSE, "Unwired?"=FALSE}, {"Label"="PNG Compression Level", "Tag"="180.1.a.Printing:PNG Compression Level", "Property Type"=enum."Base", "Indent"=1, "Can Read?"=TRUE, "Can Write?"=TRUE, "Is Read?"=FALSE, "Is Write?"=FALSE, "Inactive Parent?"=FALSE, "Unwired?"=FALSE}, {"Label"="Project", "Tag"="181.2.92.Project", "Property Type"=enum."Base", "Indent"=0, "Can Read?"=FALSE, "Can Write?"=FALSE, "Is Read?"=FALSE, "Is Write?"=FALSE, "Inactive Parent?"=TRUE, "Unwired?"=FALSE}, {"Label"="Active Project", "Tag"="181.2.92.Project:Active Project", "Property Type"=enum."Scripting", "Indent"=1, "Can Read?"=TRUE, "Can Write?"=FALSE, "Is Read?"=FALSE, "Is Write?"=FALSE, "Inactive Parent?"=FALSE, "Unwired?"=FALSE}, {"Label"="Default Project", "Tag"="182.3.81.Project:Default Project", "Property Type"=enum."Private", "Indent"=1, "Can Read?"=TRUE, "Can Write?"=FALSE, "Is Read?"=FALSE, "Is Write?"=FALSE, "Inactive Parent?"=FALSE, "Unwired?"=FALSE}, {"Label"="Get Last Max Load Time", "Tag"="183.3.87.Project:Get Last Max Load Time", "Property Type"=enum."Private", "Indent"=1, "Can Read?"=TRUE, "Can Write?"=FALSE, "Is Read?"=FALSE, "Is Write?"=FALSE, "Inactive Parent?"=FALSE, "Unwired?"=FALSE}, {"Label"="Has Any Project Been Created", "Tag"="184.3.82.Project:Has Any Project Been Created", "Property Type"=enum."Private", "Indent"=1, "Can Read?"=TRUE, "Can Write?"=FALSE, "Is Read?"=FALSE, "Is Write?"=FALSE, "Inactive Parent?"=FALSE, "Unwired?"=FALSE}, {"Label"="Libraries[]", "Tag"="185.3.88.Project:Libraries[]", "Property Type"=enum."Private", "Indent"=1, "Can Read?"=TRUE, "Can Write?"=FALSE, "Is Read?"=FALSE, "Is Write?"=FALSE, "Inactive Parent?"=FALSE, "Unwired?"=FALSE}, {"Label"="Owning Project", "Tag"="186.2.7e.Project:Owning Project", "Property Type"=enum."Scripting", "Indent"=1, "Can Read?"=TRUE, "Can Write?"=FALSE, "Is Read?"=FALSE, "Is Write?"=FALSE, "Inactive Parent?"=FALSE, "Unwired?"=FALSE}, {"Label"="Projects[]", "Tag"="187.1.69.Project:Projects[]", "Property Type"=enum."Base", "Indent"=1, "Can Read?"=TRUE, "Can Write?"=FALSE, "Is Read?"=FALSE, "Is Write?"=FALSE, "Inactive Parent?"=FALSE, "Unwired?"=FALSE}, {"Label"="Show Path in Project Window", "Tag"="188.3.85.Project:Show Path in Project Window", "Property Type"=enum."Private", "Indent"=1, "Can Read?"=TRUE, "Can Write?"=TRUE, "Is Read?"=FALSE, "Is Write?"=FALSE, "Inactive Parent?"=FALSE, "Unwired?"=FALSE}, {"Label"="Target Item", "Tag"="189.1.86.Project:Target Item", "Property Type"=enum."Base", "Indent"=1, "Can Read?"=TRUE, "Can Write?"=FALSE, "Is Read?"=FALSE, "Is Write?"=FALSE, "Inactive Parent?"=FALSE, "Unwired?"=FALSE}, {"Label"="Remote Panel", "Tag"="190.1.41.Remote Panel", "Property Type"=enum."Base", "Indent"=0, "Can Read?"=FALSE, "Can Write?"=FALSE, "Is Read?"=FALSE, "Is Write?"=FALSE, "Inactive Parent?"=TRUE, "Unwired?"=FALSE}, {"Label"="Connections To Clients", "Tag"="190.1.41.Remote Panel:Connections To Clients", "Property Type"=enum."Base", "Indent"=1, "Can Read?"=TRUE, "Can Write?"=FALSE, "Is Read?"=FALSE, "Is Write?"=FALSE, "Inactive Parent?"=FALSE, "Unwired?"=FALSE}, {"Label"="Connections To Servers", "Tag"="191.1.42.Remote Panel:Connections To Servers", "Property Type"=enum."Base", "Indent"=1, "Can Read?"=TRUE, "Can Write?"=FALSE, "Is Read?"=FALSE, "Is Write?"=FALSE, "Inactive Parent?"=FALSE, "Unwired?"=FALSE}, {"Label"="Is Supported", "Tag"="192.3.5e.Remote Panel:Is Supported", "Property Type"=enum."Private", "Indent"=1, "Can Read?"=TRUE, "Can Write?"=FALSE, "Is Read?"=FALSE, "Is Write?"=FALSE, "Inactive Parent?"=FALSE, "Unwired?"=FALSE}, {"Label"="NetLoad Monitor Enabled", "Tag"="193.3.43.Remote Panel:NetLoad Monitor Enabled", "Property Type"=enum."Private", "Indent"=1, "Can Read?"=TRUE, "Can Write?"=TRUE, "Is Read?"=FALSE, "Is Write?"=FALSE, "Inactive Parent?"=FALSE, "Unwired?"=FALSE}, {"Label"="Run Reserve XInterface Components", "Tag"="194.3.9f.Run Reserve XInterface Components", "Property Type"=enum."Private", "Indent"=0, "Can Read?"=TRUE, "Can Write?"=TRUE, "Is Read?"=FALSE, "Is Write?"=FALSE, "Inactive Parent?"=FALSE, "Unwired?"=FALSE}, {"Label"="Save for Previous", "Tag"="195.3.9d.Save for Previous", "Property Type"=enum."Base", "Indent"=0, "Can Read?"=FALSE, "Can Write?"=FALSE, "Is Read?"=FALSE, "Is Write?"=FALSE, "Inactive Parent?"=TRUE, "Unwired?"=FALSE}, {"Label"="Original App", "Tag"="195.3.9d.Save for Previous:Original App", "Property Type"=enum."Private", "Indent"=1, "Can Read?"=TRUE, "Can Write?"=FALSE, "Is Read?"=FALSE, "Is Write?"=FALSE, "Inactive Parent?"=FALSE, "Unwired?"=FALSE}, {"Label"="Separate Compiled Code For New Files", "Tag"="196.3.fb.Separate Compiled Code For New Files", "Property Type"=enum."Private", "Indent"=0, "Can Read?"=TRUE, "Can Write?"=FALSE, "Is Read?"=FALSE, "Is Write?"=FALSE, "Inactive Parent?"=FALSE, "Unwired?"=FALSE}, {"Label"="Server", "Tag"="197.1.27.Server", "Property Type"=enum."Base", "Indent"=0, "Can Read?"=FALSE, "Can Write?"=FALSE, "Is Read?"=FALSE, "Is Write?"=FALSE, "Inactive Parent?"=TRUE, "Unwired?"=FALSE}, {"Label"="Logging Enabled", "Tag"="197.1.27.Server:Logging Enabled", "Property Type"=enum."Base", "Indent"=1, "Can Read?"=TRUE, "Can Write?"=TRUE, "Is Read?"=FALSE, "Is Write?"=FALSE, "Inactive Parent?"=FALSE, "Unwired?"=FALSE}, {"Label"="Logging File Path", "Tag"="198.1.28.Server:Logging File Path", "Property Type"=enum."Base", "Indent"=1, "Can Read?"=TRUE, "Can Write?"=TRUE, "Is Read?"=FALSE, "Is Write?"=FALSE, "Inactive Parent?"=FALSE, "Unwired?"=FALSE}, {"Label"="Port", "Tag"="199.1.5d.Server:Port", "Property Type"=enum."Base", "Indent"=1, "Can Read?"=TRUE, "Can Write?"=TRUE, "Is Read?"=FALSE, "Is Write?"=FALSE, "Inactive Parent?"=FALSE, "Unwired?"=FALSE}, {"Label"="Service Name", "Tag"="200.1.94.Server:Service Name", "Property Type"=enum."Base", "Indent"=1, "Can Read?"=TRUE, "Can Write?"=TRUE, "Is Read?"=FALSE, "Is Write?"=FALSE, "Inactive Parent?"=FALSE, "Unwired?"=FALSE}, {"Label"="TCP Listener Active", "Tag"="201.1.20.Server:TCP Listener Active", "Property Type"=enum."Base", "Indent"=1, "Can Read?"=TRUE, "Can Write?"=TRUE, "Is Read?"=FALSE, "Is Write?"=FALSE, "Inactive Parent?"=FALSE, "Unwired?"=FALSE}, {"Label"="TCP/IP Access List", "Tag"="202.1.1b.Server:TCP/IP Access List", "Property Type"=enum."Base", "Indent"=1, "Can Read?"=TRUE, "Can Write?"=TRUE, "Is Read?"=FALSE, "Is Write?"=FALSE, "Inactive Parent?"=FALSE, "Unwired?"=FALSE}, {"Label"="VI Access List", "Tag"="203.1.1a.Server:VI Access List", "Property Type"=enum."Base", "Indent"=1, "Can Read?"=TRUE, "Can Write?"=TRUE, "Is Read?"=FALSE, "Is Write?"=FALSE, "Inactive Parent?"=FALSE, "Unwired?"=FALSE}, {"Label"="Source Control", "Tag"="204.3.6e.Source Control", "Property Type"=enum."Base", "Indent"=0, "Can Read?"=FALSE, "Can Write?"=FALSE, "Is Read?"=FALSE, "Is Write?"=FALSE, "Inactive Parent?"=TRUE, "Unwired?"=FALSE}, {"Label"="Configuration Data", "Tag"="204.3.6e.Source Control:Configuration Data", "Property Type"=enum."Private", "Indent"=1, "Can Read?"=TRUE, "Can Write?"=TRUE, "Is Read?"=FALSE, "Is Write?"=FALSE, "Inactive Parent?"=FALSE, "Unwired?"=FALSE}, {"Label"="Display Only Selected Files", "Tag"="205.3.71.Source Control:Display Only Selected Files", "Property Type"=enum."Private", "Indent"=1, "Can Read?"=TRUE, "Can Write?"=TRUE, "Is Read?"=FALSE, "Is Write?"=FALSE, "Inactive Parent?"=FALSE, "Unwired?"=FALSE}, {"Label"="Display Warning If File Is Checked Out", "Tag"="206.3.74.Source Control:Display Warning If File Is Checked Out", "Property Type"=enum."Private", "Indent"=1, "Can Read?"=TRUE, "Can Write?"=TRUE, "Is Read?"=FALSE, "Is Write?"=FALSE, "Inactive Parent?"=FALSE, "Unwired?"=FALSE}, {"Label"="Include InstrLib In Get Dependents", "Tag"="207.3.9c.Source Control:Include InstrLib In Get Dependents", "Property Type"=enum."Private", "Indent"=1, "Can Read?"=TRUE, "Can Write?"=TRUE, "Is Read?"=FALSE, "Is Write?"=FALSE, "Inactive Parent?"=FALSE, "Unwired?"=FALSE}, {"Label"="Include VILib In Get Dependents", "Tag"="208.3.9b.Source Control:Include VILib In Get Dependents", "Property Type"=enum."Private", "Indent"=1, "Can Read?"=TRUE, "Can Write?"=TRUE, "Is Read?"=FALSE, "Is Write?"=FALSE, "Inactive Parent?"=FALSE, "Unwired?"=FALSE}, {"Label"="Prompt to Add to SCC When Adding to Project", "Tag"="209.3.77.Source Control:Prompt to Add to SCC When Adding to Project", "Property Type"=enum."Private", "Indent"=1, "Can Read?"=TRUE, "Can Write?"=TRUE, "Is Read?"=FALSE, "Is Write?"=FALSE, "Inactive Parent?"=FALSE, "Unwired?"=FALSE}, {"Label"="Prompt to Check Out", "Tag"="210.3.76.Source Control:Prompt to Check Out", "Property Type"=enum."Private", "Indent"=1, "Can Read?"=TRUE, "Can Write?"=TRUE, "Is Read?"=FALSE, "Is Write?"=FALSE, "Inactive Parent?"=FALSE, "Unwired?"=FALSE}, {"Label"="Provider Location", "Tag"="211.3.70.Source Control:Provider Location", "Property Type"=enum."Private", "Indent"=1, "Can Read?"=TRUE, "Can Write?"=TRUE, "Is Read?"=FALSE, "Is Write?"=FALSE, "Inactive Parent?"=FALSE, "Unwired?"=FALSE}, {"Label"="Provider Name", "Tag"="212.3.6f.Source Control:Provider Name", "Property Type"=enum."Private", "Indent"=1, "Can Read?"=TRUE, "Can Write?"=TRUE, "Is Read?"=FALSE, "Is Write?"=FALSE, "Inactive Parent?"=FALSE, "Unwired?"=FALSE}, {"Label"="Select Callers When Checking Files Out", "Tag"="213.3.73.Source Control:Select Callers When Checking Files Out", "Property Type"=enum."Private", "Indent"=1, "Can Read?"=TRUE, "Can Write?"=TRUE, "Is Read?"=FALSE, "Is Write?"=FALSE, "Inactive Parent?"=FALSE, "Unwired?"=FALSE}, {"Label"="Select Hierarchy When Adding Files", "Tag"="214.3.72.Source Control:Select Hierarchy When Adding Files", "Property Type"=enum."Private", "Indent"=1, "Can Read?"=TRUE, "Can Write?"=TRUE, "Is Read?"=FALSE, "Is Write?"=FALSE, "Inactive Parent?"=FALSE, "Unwired?"=FALSE}, {"Label"="Use Dialog Box For File Checkout", "Tag"="215.3.75.Source Control:Use Dialog Box For File Checkout", "Property Type"=enum."Private", "Indent"=1, "Can Read?"=TRUE, "Can Write?"=TRUE, "Is Read?"=FALSE, "Is Write?"=FALSE, "Inactive Parent?"=FALSE, "Unwired?"=FALSE}, {"Label"="Statechart", "Tag"="216.3.b7.Statechart", "Property Type"=enum."Base", "Indent"=0, "Can Read?"=FALSE, "Can Write?"=FALSE, "Is Read?"=FALSE, "Is Write?"=FALSE, "Inactive Parent?"=TRUE, "Unwired?"=FALSE}, {"Label"="CodeGenCaseStruct", "Tag"="216.3.b7.Statechart:CodeGenCaseStruct", "Property Type"=enum."Private", "Indent"=1, "Can Read?"=TRUE, "Can Write?"=TRUE, "Is Read?"=FALSE, "Is Write?"=FALSE, "Inactive Parent?"=FALSE, "Unwired?"=FALSE}, {"Label"="InlineTopLevelGraph", "Tag"="217.3.bd.Statechart:InlineTopLevelGraph", "Property Type"=enum."Private", "Indent"=1, "Can Read?"=TRUE, "Can Write?"=TRUE, "Is Read?"=FALSE, "Is Write?"=FALSE, "Inactive Parent?"=FALSE, "Unwired?"=FALSE}, {"Label"="Is Installed", "Tag"="218.3.ee.Statechart:Is Installed", "Property Type"=enum."Private", "Indent"=1, "Can Read?"=TRUE, "Can Write?"=FALSE, "Is Read?"=FALSE, "Is Write?"=FALSE, "Inactive Parent?"=FALSE, "Unwired?"=FALSE}, {"Label"="Show Configuration", "Tag"="219.3.b4.Statechart:Show Configuration", "Property Type"=enum."Private", "Indent"=1, "Can Read?"=TRUE, "Can Write?"=FALSE, "Is Read?"=FALSE, "Is Write?"=FALSE, "Inactive Parent?"=FALSE, "Unwired?"=FALSE}, {"Label"="Show Custom Icon", "Tag"="220.3.b3.Statechart:Show Custom Icon", "Property Type"=enum."Private", "Indent"=1, "Can Read?"=TRUE, "Can Write?"=FALSE, "Is Read?"=FALSE, "Is Write?"=FALSE, "Inactive Parent?"=FALSE, "Unwired?"=FALSE}, {"Label"="Show Path for IsIn", "Tag"="221.3.b8.Statechart:Show Path for IsIn", "Property Type"=enum."Private", "Indent"=1, "Can Read?"=TRUE, "Can Write?"=FALSE, "Is Read?"=FALSE, "Is Write?"=FALSE, "Inactive Parent?"=FALSE, "Unwired?"=FALSE}, {"Label"="Suppress Auto Update Dependencies", "Tag"="222.3.a9.Suppress Auto Update Dependencies", "Property Type"=enum."Private", "Indent"=0, "Can Read?"=TRUE, "Can Write?"=TRUE, "Is Read?"=FALSE, "Is Write?"=FALSE, "Inactive Parent?"=FALSE, "Unwired?"=FALSE}, {"Label"="Supress Update Name Preflight", "Tag"="223.3.b0.Supress Update Name Preflight", "Property Type"=enum."Private", "Indent"=0, "Can Read?"=TRUE, "Can Write?"=TRUE, "Is Read?"=FALSE, "Is Write?"=FALSE, "Inactive Parent?"=FALSE, "Unwired?"=FALSE}, {"Label"="Tool Number", "Tag"="224.3.ae.Tool Number", "Property Type"=enum."Private", "Indent"=0, "Can Read?"=TRUE, "Can Write?"=TRUE, "Is Read?"=FALSE, "Is Write?"=FALSE, "Inactive Parent?"=FALSE, "Unwired?"=FALSE}, {"Label"="VIObjCache", "Tag"="225.3.f3.VIObjCache", "Property Type"=enum."Base", "Indent"=0, "Can Read?"=FALSE, "Can Write?"=FALSE, "Is Read?"=FALSE, "Is Write?"=FALSE, "Inactive Parent?"=TRUE, "Unwired?"=FALSE}, {"Label"="Available in RTE", "Tag"="225.3.f3.VIObjCache:Available in RTE", "Property Type"=enum."Private", "Indent"=1, "Can Read?"=TRUE, "Can Write?"=TRUE, "Is Read?"=FALSE, "Is Write?"=FALSE, "Inactive Parent?"=FALSE, "Unwired?"=FALSE}, {"Label"="DistPath", "Tag"="226.3.f7.VIObjCache:DistPath", "Property Type"=enum."Private", "Indent"=1, "Can Read?"=TRUE, "Can Write?"=FALSE, "Is Read?"=FALSE, "Is Write?"=FALSE, "Inactive Parent?"=FALSE, "Unwired?"=FALSE}, {"Label"="UserPath", "Tag"="227.3.f8.VIObjCache:UserPath", "Property Type"=enum."Private", "Indent"=1, "Can Read?"=TRUE, "Can Write?"=FALSE, "Is Read?"=FALSE, "Is Write?"=FALSE, "Inactive Parent?"=FALSE, "Unwired?"=FALSE}, {"Label"="Web Server", "Tag"="228.1.b5.Web Server", "Property Type"=enum."Base", "Indent"=0, "Can Read?"=FALSE, "Can Write?"=FALSE, "Is Read?"=FALSE, "Is Write?"=FALSE, "Inactive Parent?"=TRUE, "Unwired?"=FALSE}, {"Label"="Config File Path", "Tag"="228.1.b5.Web Server:Config File Path", "Property Type"=enum."Base", "Indent"=1, "Can Read?"=TRUE, "Can Write?"=FALSE, "Is Read?"=FALSE, "Is Write?"=FALSE, "Inactive Parent?"=FALSE, "Unwired?"=FALSE}, {"Label"="Default Config File Path", "Tag"="229.1.b6.Web Server:Default Config File Path", "Property Type"=enum."Base", "Indent"=1, "Can Read?"=TRUE, "Can Write?"=FALSE, "Is Read?"=FALSE, "Is Write?"=FALSE, "Inactive Parent?"=FALSE, "Unwired?"=FALSE}, {"Label"="HTTP Port", "Tag"="230.1.30.Web Server:HTTP Port", "Property Type"=enum."Base", "Indent"=1, "Can Read?"=TRUE, "Can Write?"=TRUE, "Is Read?"=FALSE, "Is Write?"=FALSE, "Inactive Parent?"=FALSE, "Unwired?"=FALSE}, {"Label"="Logging Enabled", "Tag"="231.1.32.Web Server:Logging Enabled", "Property Type"=enum."Base", "Indent"=1, "Can Read?"=TRUE, "Can Write?"=TRUE, "Is Read?"=FALSE, "Is Write?"=FALSE, "Inactive Parent?"=FALSE, "Unwired?"=FALSE}, {"Label"="Logging File Path", "Tag"="232.1.33.Web Server:Logging File Path", "Property Type"=enum."Base", "Indent"=1, "Can Read?"=TRUE, "Can Write?"=TRUE, "Is Read?"=FALSE, "Is Write?"=FALSE, "Inactive Parent?"=FALSE, "Unwired?"=FALSE}, {"Label"="Read Timeout", "Tag"="233.1.31.Web Server:Read Timeout", "Property Type"=enum."Base", "Indent"=1, "Can Read?"=TRUE, "Can Write?"=TRUE, "Is Read?"=FALSE, "Is Write?"=FALSE, "Inactive Parent?"=FALSE, "Unwired?"=FALSE}, {"Label"="Root Directory Path", "Tag"="234.1.2f.Web Server:Root Directory Path", "Property Type"=enum."Base", "Indent"=1, "Can Read?"=TRUE, "Can Write?"=TRUE, "Is Read?"=FALSE, "Is Write?"=FALSE, "Inactive Parent?"=FALSE, "Unwired?"=FALSE}, {"Label"="Server Active", "Tag"="235.1.2e.Web Server:Server Active", "Property Type"=enum."Base", "Indent"=1, "Can Read?"=TRUE, "Can Write?"=TRUE, "Is Read?"=FALSE, "Is Write?"=FALSE, "Inactive Parent?"=FALSE, "Unwired?"=FALSE}, {"Label"="TCP/IP Access List", "Tag"="236.1.34.Web Server:TCP/IP Access List", "Property Type"=enum."Base", "Indent"=1, "Can Read?"=TRUE, "Can Write?"=TRUE, "Is Read?"=FALSE, "Is Write?"=FALSE, "Inactive Parent?"=FALSE, "Unwired?"=FALSE}, {"Label"="VI Access List", "Tag"="237.1.35.Web Server:VI Access List", "Property Type"=enum."Base", "Indent"=1, "Can Read?"=TRUE, "Can Write?"=TRUE, "Is Read?"=FALSE, "Is Write?"=FALSE, "Inactive Parent?"=FALSE, "Unwired?"=FALSE}]
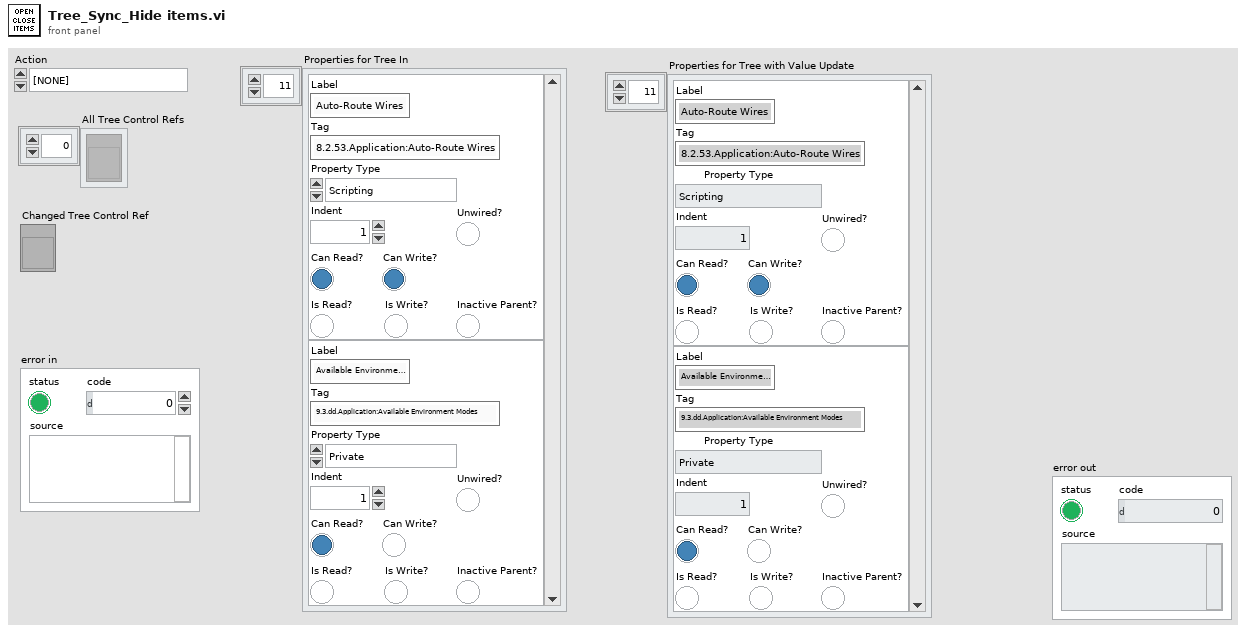
[diagram p1: front panel]
types:
  T1 = cluster{"Label":string, "Tag":string, "Property Type":enum16{"Unknown", "Base", "Scripting", "Private", "Deprecated", "None", "Divider"}, "Indent":u16, "Can Read?":bool, "Can Write?":bool, "Is Read?":bool, "Is Write?":bool, "Inactive Parent?":bool, "Unwired?":bool}[]
  T2 = typedef "action enum.ctl" = enum16{"[NONE]", "Wire Bundle", "Wire Unbundle", "Terminal Unbundle", "Terminal Bundle", "Bundler Move Up", "Bundler Move Down", "Bundler Insert", "Bundler Remove", "Bundler Remove Unwired", "Bundler Rearrange", "In Place Insert", "In Place Remove", "In Place Remove Unwired", "In Place Rearrange", "Wire Properties", "Wire Method", "Terminal Properties", "Terminal Method", "Property Move Up", "Property Move Down", "Properties Insert", "Properties Remove", "Properties Remove Unwired", "Properties Rearrange", "Method Change", "Class for Constant", "Class For Control", "Class For Node", "Class Name to Clipboard"}
  T3 = cluster{"Label":string, "Tag":string, "Property Type":enum16{"Unknown", "Base", "Scripting", "Private", "Deprecated", "None", "Divider"}, "Indent":u16, "Can Read?":bool, "Can Write?":bool, "Is Read?":bool, "Is Write?":bool, "Inactive Parent?":bool, "Unwired?":bool}
  T4 = cluster{"Left Cell String":string, "Child Text":string[], "Child Tag":string, "Item Indent":i32, "Child Only?":bool, "Glyph Index":i32}[]
  T5 = typedef "LVNodeAndColumnTypeDef.ctl" = cluster{"Node":string, "Column":i32}
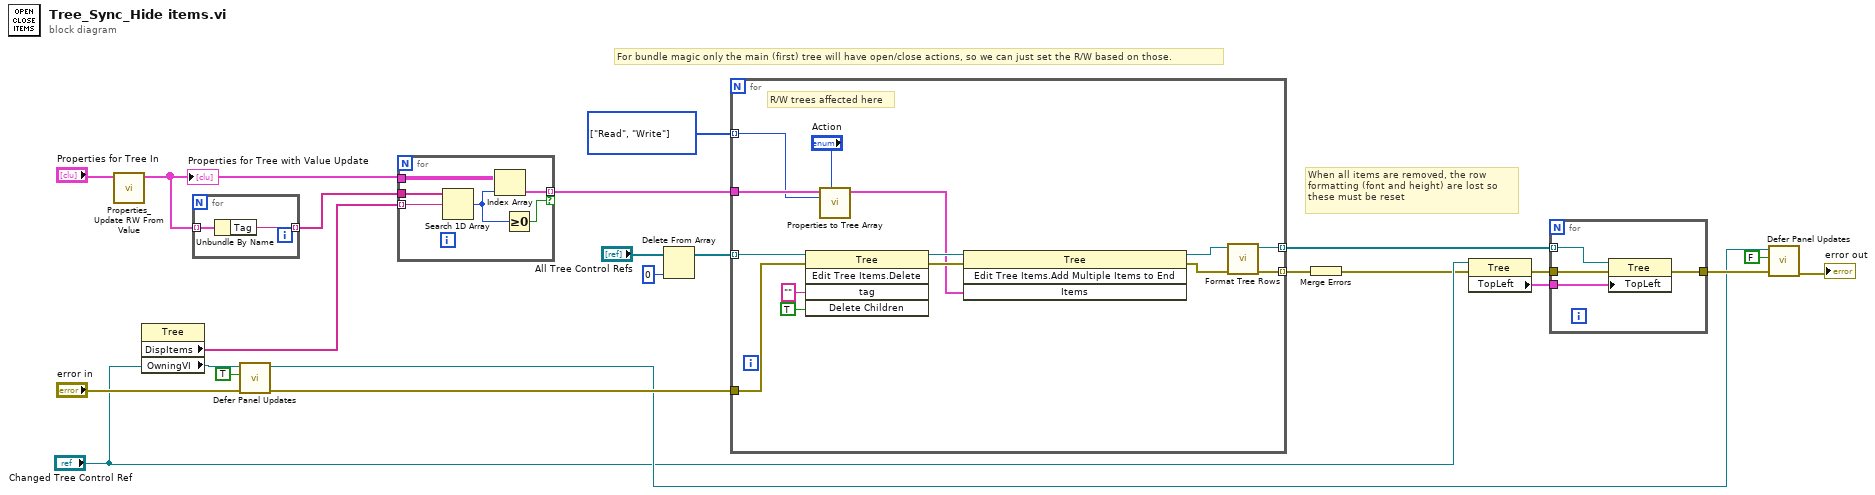
[diagram p0: block diagram]
diagram:
  w7 = enum16{"Main", "Write", "Read"}[] [enum."Read", enum."Write"] items=["Main", "Write", "Read"] ("Tree Type")
  # "When all items are removed, the row formatting (font and height) are lost so these must be reset"
  # "For bundle magic only the main (first) tree will have open/close actions, so we can just set the R/W based on those."
  n1 = call "Properties_Update RW From Value.vi"("Properties for Tree In"="Properties for Tree In") -> ("Properties for Tree Out"=w8:T1)  [unwired: 10 in]
  "Properties for Tree with Value Update" <- w8
  n2 = property class="Tree"(reference="Changed Tree Control Ref") -> ("DispItems"=w20:string[], "OwningVI"=w13:refnum<vi>)  [unwired: 1 in, 2 out]
  n3 = for {
    tunnel: w8 -> [w25] mode=indexing
    tunnel: [w24] -> w19 mode=indexing
    n4 = Unbundle By Name(w25) -> ("Tag"=w24:string)
  }
  n5 = call "Defer Panel Updates.vi"("error in (no error)"="error in", "Defer Panel Updates [T]"=TRUE, "VI Ref"=w13) -> ("error out"=w15:errorcluster, "VI Ref Out"=w12:refnum<vi>)  [unwired: 7 in]
  n6 = for {
    tunnel: w8 -> [w29]
    tunnel: w19 -> [w30]
    tunnel: w20 -> [w31] mode=indexing
    tunnel: [w28] -> w3 mode=indexing if=w26
    n7 = Search 1D Array(1D array=w30, element=w31) -> (index of element=w27:i32)  [unwired: 1 in]
    n8 = Index Array(array=w29, index=w27) -> (element=w28:T3)
    n9 = Greater Or Equal To 0?(x=w27) -> (x >= 0?=w26:bool)
  }
  n10 = Delete From Array(array="All Tree Control Refs", index=0) -> (array with subset deleted=w21:refnum<vi>[])  [unwired: 1 in, 1 out]
  n11 = for {
    tunnel: w21 -> [w45] mode=indexing
    tunnel: w15 -> [w44]
    tunnel: [w32] -> w5 mode=indexing
    tunnel: w7 -> [w37] mode=indexing
    tunnel: w3 -> [w38]
    tunnel: [w33] -> w2 mode=indexing
    # "R/W trees affected here"
    n12 = invoke class="Tree" method="Edit Tree Items.Delete"(reference=w45, error in=w44, "tag"="" ("Tag"), "Delete Children"=TRUE ("Delete Children?")) -> (reference out=w41:refnum<vi>, error out=w40:errorcluster)  [unwired: 1 in, 3 out]
    n13 = call "Properties to Tree Array.vi"("Action"="Action", "Tree Type"=w37, "Properties for Tree"=w38) -> ("Tree Arr"=w39:T4)  [unwired: 8 in]
    n14 = invoke class="Tree" method="Edit Tree Items.Add Multiple Items to End"(reference=w41, error in=w40, "Items"=w39) -> (reference out=w34:refnum<vi>, error out=w35:errorcluster)  [unwired: 1 in, 2 out]
    n15 = call "Format Tree Rows.vi"("error in"=w35, "Tree Ref"=w34) -> ("error out"=w32:errorcluster, "Tree Ref out"=w33:refnum<vi>)  [unwired: 8 in]
  }
  n16 = Merge Errors(w5) -> (w1:errorcluster)
  n17 = property class="Tree"(reference="Changed Tree Control Ref", error in=w1) -> (error out=w4:errorcluster, "TopLeft"=w10:T5)  [unwired: 1 out]
  n18 = for {
    tunnel: w2 -> [w47] mode=indexing
    tunnel: [w48] -> w18
    tunnel: w10 -> [w49]
    tunnel: w4 -> [w46]
    n19 = property class="Tree"(reference=w47, error in=w46, "TopLeft"=w49) -> (error out=w48:errorcluster)  [unwired: 1 out]
  }
  n20 = call "Defer Panel Updates.vi"("error in (no error)"=w18, "Defer Panel Updates [T]"=FALSE, "VI Ref"=w12) -> ("error out"=→"error out":errorcluster)  [unwired: 7 in, 1 out]
